vi "GUI_Cameras.vi"(1 "GUIdevice 1":string="HPD_CCD") -> (0 "Image (IMAQ)":T1(plugin-control))   [LabVIEW 2013]
uses:
  Shared/GUI_Template/GUI_master/tcp_new_data_event.ctl
  Shared/GUI_Template/GUI_master/tcp new data cluster.ctl
  color tables/image color table presets.ctl
  Controls/Crosshair type def.ctl
  Controls/IMAQ control.ctl
  <vilib>/vision/Image Controls.llb/IMAQ Image.ctl
  Controls/Image Processing Controls.ctl
  Controls/GUI_running average centroid overlay.ctl
  Controls/Image Analysis Controls.ctl
  <vilib>/Utility/miscctls.llb/LVRectTypeDef.ctl
  <userlib>/_OpenG.lib/comparison/comparison.llb/Boolean Changed__ogtk.vi
  <vilib>/vision/NI_Vision_Development_Module.lvlib
panel:
  in  "stop":bool
  in  "Maximize!!":bool
  out "image::1":T1(plugin-control) caption="HPD_CCD"
  out "tcp data event":T2
  in  "Tab Control":T3(tab)
  in  "Max count":T4(ring)
  in  "Size & Tolerance":T5={"X Size"=5, "Y Size"=5, "% Tolerance"=100} {"Y Size" min=1 max=8; "X Size" min=1 max=8}
  in  "Clear ROI":bool caption="draw Xhair"
  in  "Set ROI":bool caption="draw Xhair"
  in  "LowPass":bool
  out "Max Counts":dbl(slide) scale=0.0..256.0
  in  "Color table":T6
  out "Rate (Hz)":sgl
  in  "analysis::1":bool caption="Analysis"
  in  "Scale":bool
  in  "Autoscale":bool
  in  "trigger::1":bool caption="Trigger"
  in  "save::1":bool caption="Save"
  in  "Beep If Sat.":bool
  in  "roi.offsetY::1":u32 caption="ROI:OffsetY" max=1000
  in  "roi.offsetX::1":u32 caption="ROI:OffsetX" max=1288
  in  "roi.height::1":u32 caption="ROI:Height" min=1 max=728
  in  "roi.width::1":u32 caption="ROI.Width" min=1 max=1288
  in  "SpatialCalibration::1":dbl caption="um/pix" min=0.0 max=9999999.0
  in  "Sat Level":sgl=255.0
  in  "triggerdelay::1":dbl caption="Triggerdelay" min=0.0 max=10000000.0
  in  "exposure::1":dbl=0.52 caption="Exposure" min=1e-07 max=5.0
  in  "gain::1":dbl caption="Gain" min=0.0 max=24.0
  in  "scale factor":dbl=2.0 caption="Scale factor"
  out "UDP error message":string caption="Device Errors"
  in  "Crosshair.Label2::1":string="HPD_CCD" caption="CrosshairLabel2"
  in  "Crosshair.Label1::1":string="HPD_CCD" caption="CrosshairLabel1"
  in  "Target2.X::1":dbl caption="Target2X" min=0.0 max=2000.0
  in  "Target2.Y::1":dbl caption="Target2Y" min=0.0 max=2000.0
  in  "draw Xhair 2":bool caption="draw Xhair"
  in  "Target2Size.X::1":dbl=20.0 caption="Size2 x" min=0.0 max=2000.0
  in  "Target2Size.Y::1":dbl=20.0 caption="Size2 y" min=0.0 max=2000.0
  in  "Crosshair 2\nColor":u32(colorbox)=1250067
  in  "Crosshair 2Thickness":i32=1 caption="Crosshair 2\nThickness" min=0 max=2000
  in  "Overlay\nCentroid":T7={"draw Xhair 2"=FALSE, "Size x"=20.0, "Size y"=20.0, "# images to average"=20, "Centroid \nOverlay Color"=13435100} {"# images to average" min=0 max=2000; "Size y" min=0.0 max=2000.0; "Size x" min=0.0 max=2000.0}
  in  "GUI Crosshair":T8={"Draw"=FALSE, "Target"={"x"=0.0, "y"=0.0}, "Size"={"x"=20.0, "y"=20.0}, "Angle"=0.0, "Color"=1250067, "Thickness"=1, "CrosshairLabel"=""} {"Thickness" max=0; "Angle" format="%#_13g"; "Size"."y" min=0.0 max=0.0; "Size"."x" min=0.0 max=0.0}
  in  "Target.X::1":dbl caption="TargetX" min=0.0 max=2000.0
  in  "Target.Y::1":dbl caption="TargetY" min=0.0 max=2000.0
  in  "draw Xhair":bool=TRUE
  in  "TargetSize.X::1":dbl=20.0 caption="Size x" min=2.0 max=3000.0
  in  "TargetSize.Y::1":dbl=20.0 caption="Size y" min=2.0 max=3000.0
  in  "Crosshair\nColor":u32(colorbox)=1250067
  in  "Crosshair Thickness":i32=1 caption="Crosshair\nThickness" min=0 max=2000
  out "2ndmomW0y45::1":dbl caption="2ndmomW0y45" min=0.0 max=999999.0
  out "2ndmomW0x45::1":dbl caption="2ndmomW0x45" min=0.0 max=999999.0
  out "2ndmomW0y::1":dbl caption="2ndmomW0y" min=0.0 max=999999.0
  in  "Tab Control 2":enum32{"Mean", "Histogram", "Lineout"}(tab)
  out "Chart":dbl[][](graph)
  out "histogram":T9(graph)
  out "Mean Value":sgl format="%.2f"
  out "lineout":cluster{"x0":sgl, "dx":sgl, "Pixels Line":sgl[]}(graph)
  in  "GUI_Analysis":bool
  out "FWHMx (um)":dbl
  out "FWHMy (um)":dbl
  out "2ndmomW0x::1":dbl caption="2ndmomW0x" min=0.0 max=999999.0
  in  "FWHMx::1":dbl caption="FWHMx" min=0.0 max=999999.0
  in  "FWHMy::1":dbl caption="FWHMy" min=0.0 max=999999.0
  in  "centroidx::1":dbl caption="Centroidx" min=0.0 max=0.0
  in  "centroidy::1":dbl caption="Centroidy" min=0.0 max=0.0
  out "meancounts::1":dbl caption="MeanCounts" min=0.0 max=999999999.0
  in  "maxcounts::1":dbl caption="MaxCounts" min=0.0 max=999999999.0
  in  "localsavingpath::1":path caption="LocalSavingPath"
  in  "Hide controls":bool
  out "Current State":string
  # "Mean"
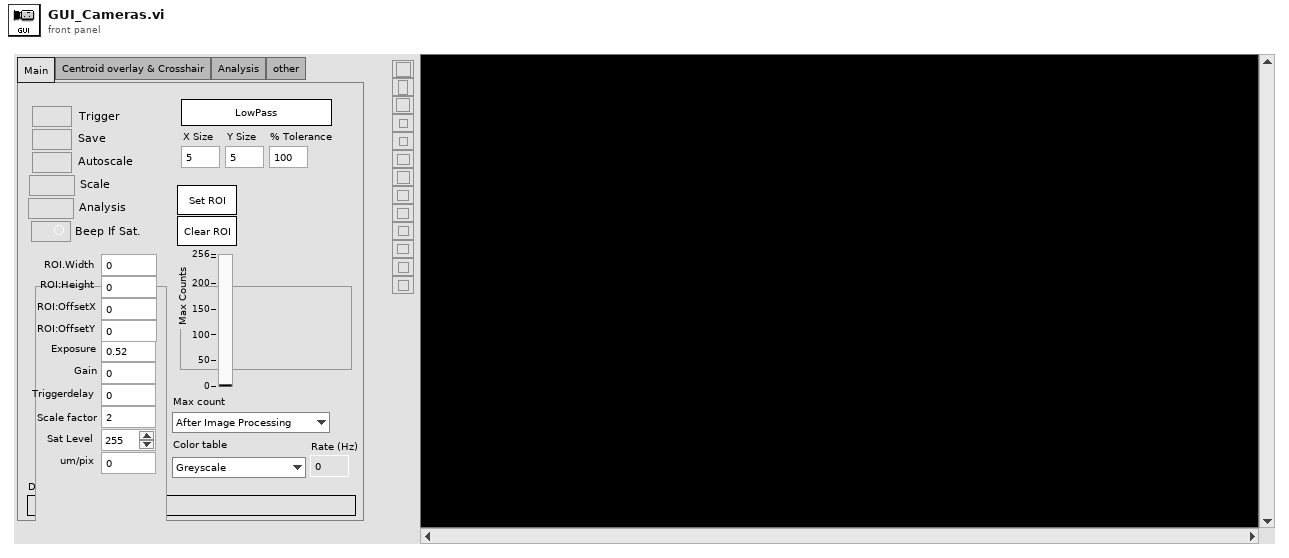
[diagram p1: front panel]
types:
  T1 = typedef "IMAQ Image.ctl" = refnum<image>
  T2 = typedef "tcp_new_data_event.ctl" = refnum<user-event>
  T3 = enum32{"Main", "Centroid overlay & Crosshair", "Analysis", "other"}
  T4 = enum16{"After Image Processing", "Before Image Processing"}
  T5 = cluster{"X Size":i32, "Y Size":i32, "% Tolerance":i32}
  T6 = typedef "image color table presets.ctl" = enum16{"Greyscale", "Binary", "Gradient", "Rainbow", "Temperature", "enhance low", "blue yellow red", "BYR enhance low", "white blue yellow", "BWR enhance low", "make a new one"}
  T7 = cluster{"draw Xhair 2":bool, "Size x":dbl, "Size y":dbl, "# images to average":i32, "Centroid \nOverlay Color":u32}
  T8 = typedef "Crosshair type def.ctl" = cluster{"Draw":bool, "Target":cluster{"x":dbl, "y":dbl}, "Size":cluster{"x":dbl, "y":dbl}, "Angle":dbl, "Color":u32, "Thickness":u8, "CrosshairLabel":string}
  T9 = cluster{"Starting Value":sgl, "Incremental Value":sgl, "Histogram":u32[]}
  T10 = enum32{"Invalid", "Standard", "Closed", "Hidden", "Minimized", "Maximized"}
  T11 = enum32{"invalid app kind", "Development System", "Run Time System", "Student Edition", "Embedded LabVIEW", "Evaluation", "Custom"}
  T12 = typedef "tcp new data cluster.ctl" = cluster{"EventEnum":enum16{"new data", "connection status update"}, "Device name":string}
  T13 = typedef "GUI_running average centroid overlay.ctl" = cluster{"CentroidX array":dbl[], "CentroidY array":dbl[], "CentroidX":dbl, "CentroidY":dbl, "# images to average":i32, "Crosshair":T8}
  T14 = cluster{"2ndmomW0y45::1":dbl, "2ndmomW0x45::1":dbl, "2ndmomW0y::1":dbl, "2ndmomW0x::1":dbl}
  T15 = cluster{"SpatialCalibration":dbl, "FWHMx":dbl, "FWHMy":dbl, "Analysis":bool}
  T16 = cluster{"LowPass":bool, "Size & Tolerance":cluster{"X Size":i32, "Y Size":i32, "% Tolerance":i32}}
  T17 = cluster{"Global Rectangle":i32[], "Contours":cluster{"Contour Type":u32, "ROI Type":u32, "Points":i32[]}[]}
  T18 = typedef "IMAQ Rectangle" = cluster{"Left":i32, "Top":i32, "Right":i32, "Bottom":i32, "Rotation":dbl}
  T19 = typedef "IMAQ control.ctl" = cluster{"Image SM":T1, "valid image":bool, "X resolution":i32, "Y resolution":i32, "Image Area":cluster{"Width":u32, "Height":u32}, "zoom to fit":bool, "Image Center":cluster{"X":u32, "Y":u32}, "Max count":dbl}
  T20 = typedef "Image Processing Controls.ctl" = cluster{"Crosshair IN":T8, "Autoscale":bool, "Scale":cluster{"scale factor":dbl, "Scale":bool}, "Lowpass IN":cluster{"LowPass":bool, "Size & Tolerance":cluster{"X Size":i32, "Y Size":i32, "% Tolerance":i32}}, "Image":T1, "GUI_centroid overlay":T13, "GUI Crosshair":T8, "Crosshair2 IN":T8}
  T21 = typedef "Image Analysis Controls.ctl" = cluster{"Analysis":cluster{"IN":cluster{"SpatialCalibration":dbl, "FWHMx":dbl, "FWHMy":dbl, "Analysis":bool}, "OUT":cluster{"FWHMx (um)":dbl, "FWHMy (um)":dbl}}, "Histogram OUT":cluster{"histogram":cluster{"Starting Value":sgl, "Incremental Value":sgl, "Histogram":u32[]}, "Mean Value Graph":sgl, "Mean Value":sgl}, "Lineout":cluster{"IN":cluster{"ROI":cluster{"Global Rectangle":i32[], "Contours":cluster{"Contour Type":u32, "ROI Type":u32, "Points":i32[]}[]}}, "OUT":cluster{"lineout":cluster{"x0":sgl, "dx":sgl, "Pixels Line":sgl[]}, "Centroid":cluster{"X Centroid":sgl, "Y Centroid":sgl}, "Max Counts":cluster{"Max":sgl, "Color":u32}}}, "Image":T1, "variables":cluster{"2ndmomW0y45::1":dbl, "2ndmomW0x45::1":dbl, "2ndmomW0y::1":dbl, "2ndmomW0x::1":dbl}}
  T22 = typedef "LVRectTypeDef.ctl" = cluster{"Left":i16, "Top":i16, "Right":i16, "Bottom":i16}
  T23 = cluster{"Core":cluster{"Current VI Reference":refnum<vi>, "Close Panel on Exit?":bool}, "tcp connections":refnum<k5>[], "subscribe messages":string[], "Image Data":T19, "Image Process":T20, "Image Analysis":T21, "FP":cluster{"size":T22, "Resize Image":bool}, "Max count":dbl, "Max count before Image Processing":dbl, "Supergui":cluster{"image::1":T1, "STOP queue":refnum<queue>, "SuperGUI ref":refnum<vi>}, "Graph":dbl[][], "New Image":T1, "All Devices":string[]}
  T24 = typedef "Image Type" = u32
  T25 = cluster{"image::1":T1, "STOP queue":refnum<queue>, "SuperGUI ref":refnum<vi>}
  T26 = cluster{"Current VI Reference":refnum<vi>, "Close Panel on Exit?":bool}
  T27 = cluster{"histogram":u32[], "Minimal Value":sgl, "Maximal Value":sgl, "Starting Value":sgl, "Interval Width":sgl, "Mean Value":sgl, "Standard  Variation":sgl, "Area (pixels)":i32}
  T28 = cluster{"TargetSize.X::1":dbl, "TargetSize.Y::1":dbl}
  T29 = cluster{"Target2Size.X::1":dbl, "Target2Size.Y::1":dbl}
  T30 = cluster{"lineout":cluster{"x0":sgl, "dx":sgl, "Pixels Line":sgl[]}, "Centroid":cluster{"X Centroid":sgl, "Y Centroid":sgl}, "Max Counts":cluster{"Max":sgl, "Color":u32}}
  T31 = cluster{"histogram":cluster{"Starting Value":sgl, "Incremental Value":sgl, "Histogram":u32[]}, "Mean Value Graph":sgl, "Mean Value":sgl}
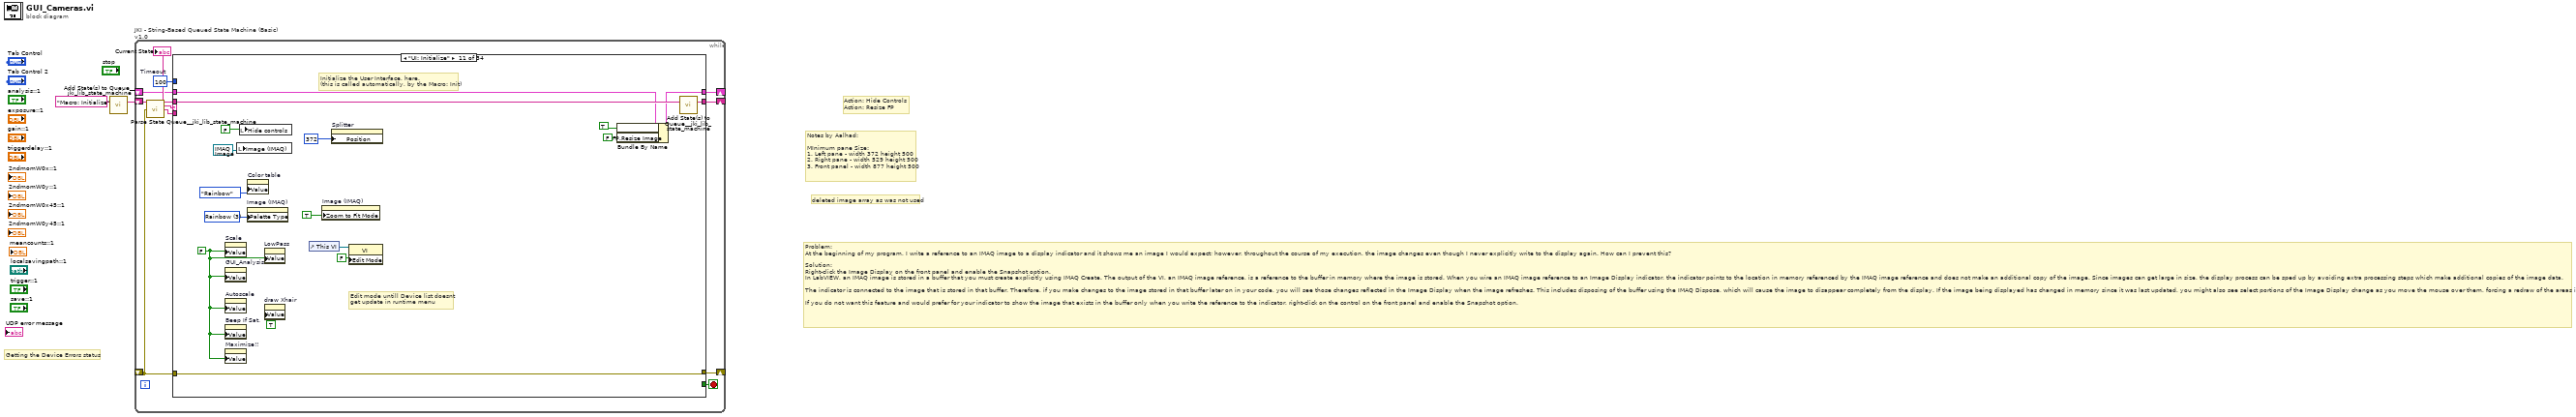
[diagram p0: block diagram]
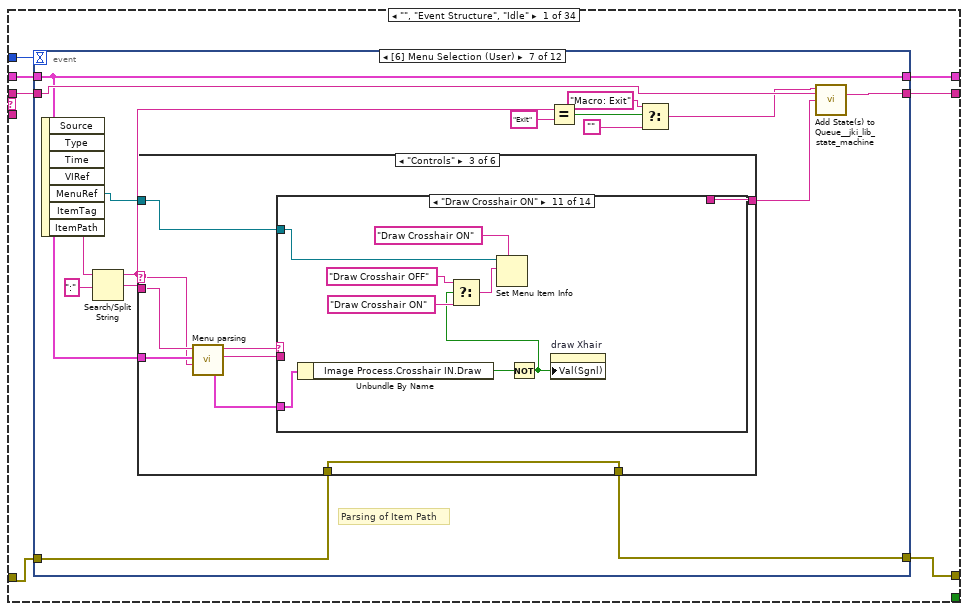
[diagram p2: hidden frame]
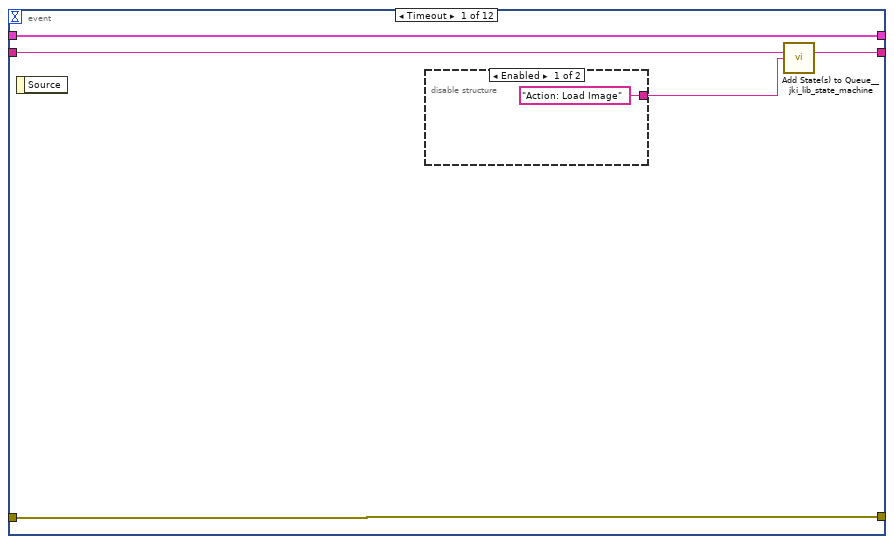
[diagram p3: hidden frame]
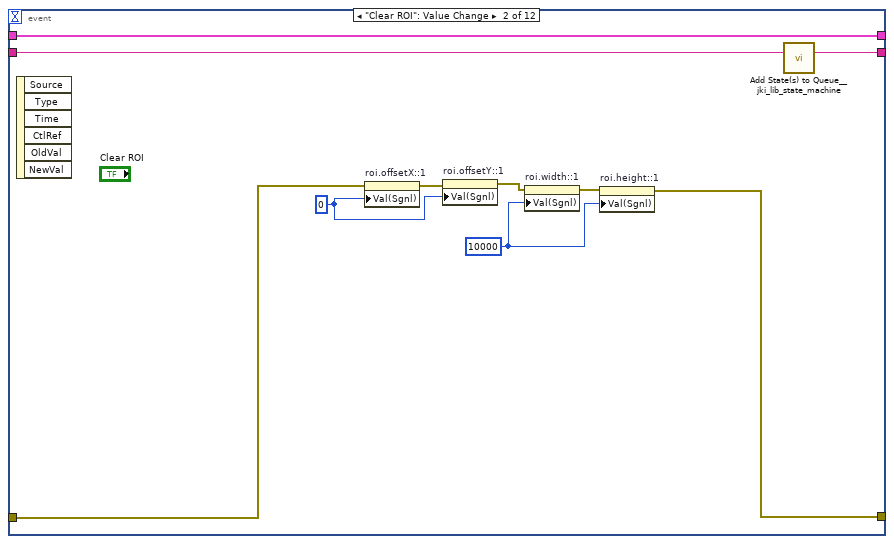
[diagram p5: hidden frame]
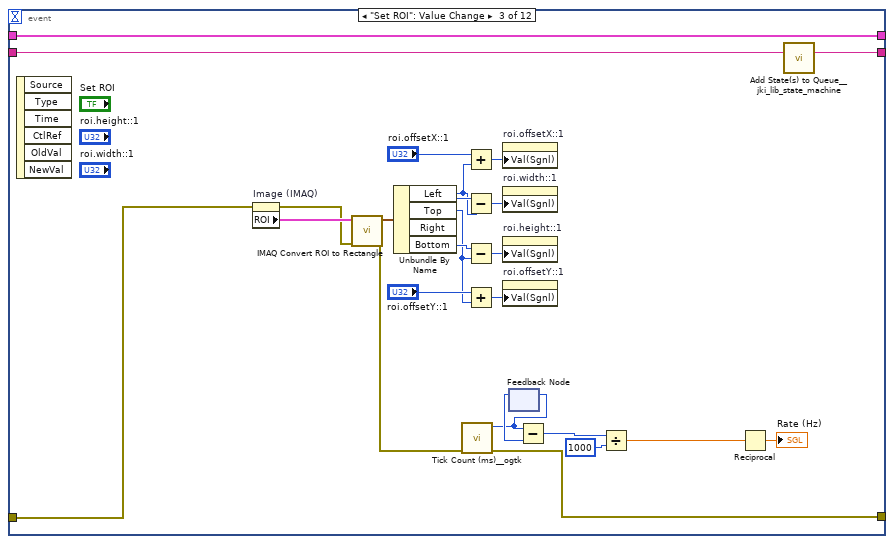
[diagram p6: hidden frame]
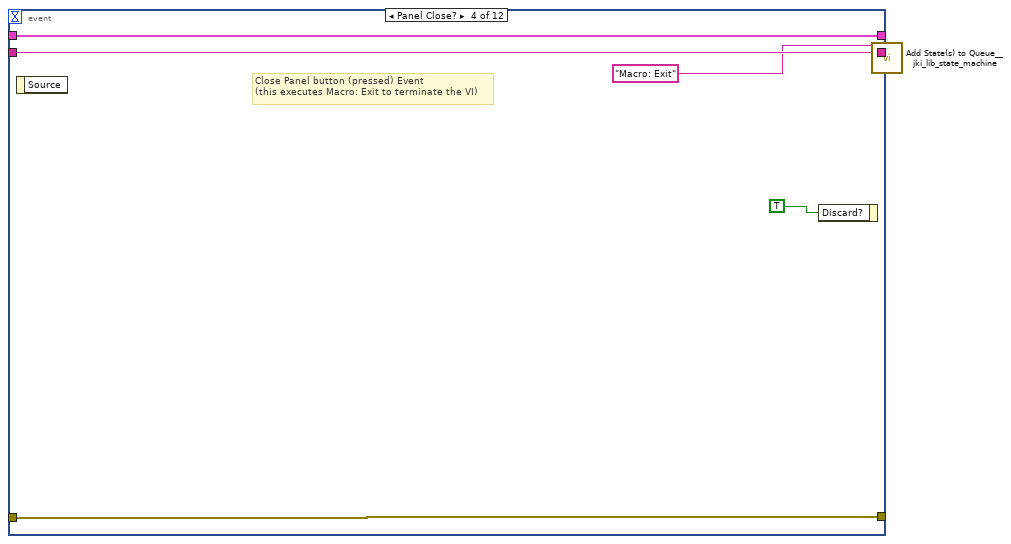
[diagram p7: hidden frame]
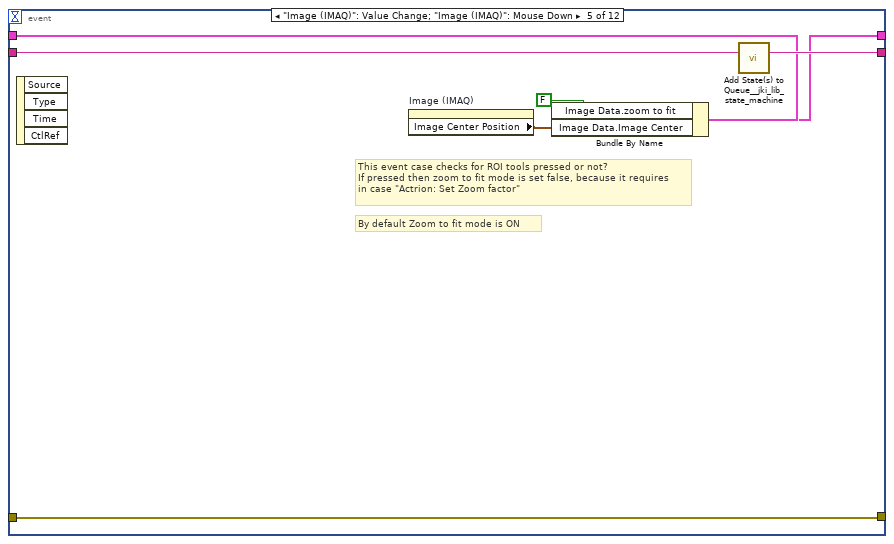
[diagram p8: hidden frame]
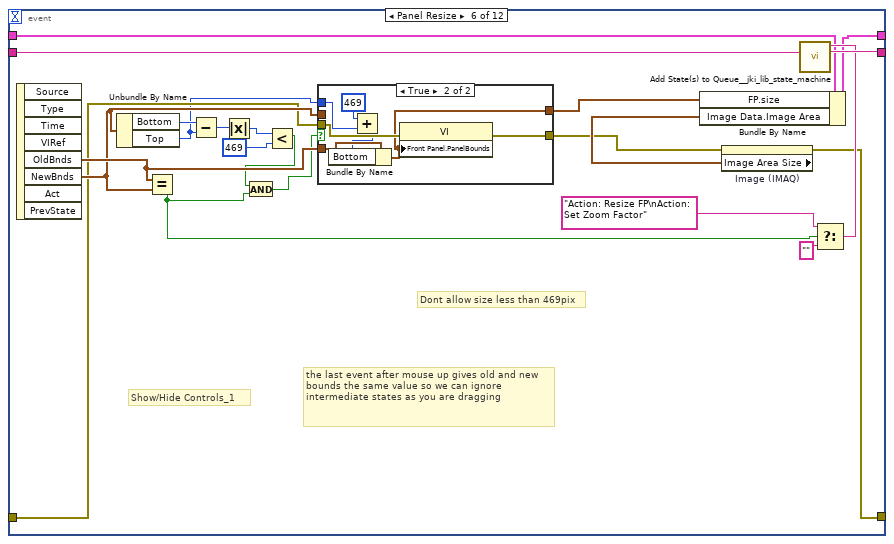
[diagram p9: hidden frame]
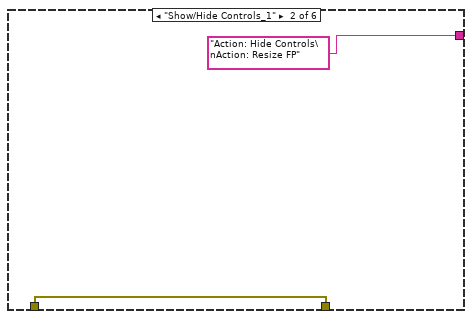
[diagram p12: hidden frame]
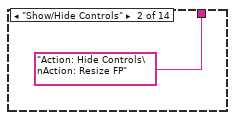
[diagram p14: hidden frame]
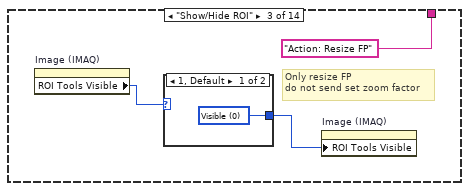
[diagram p15: hidden frame]
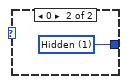
[diagram p16: hidden frame]
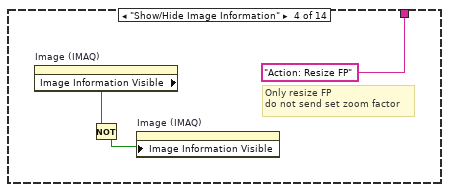
[diagram p17: hidden frame]
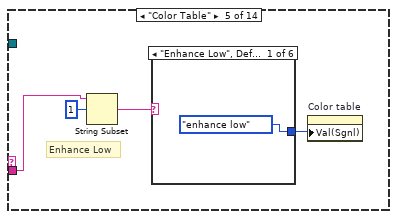
[diagram p18: hidden frame]
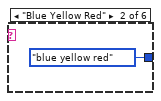
[diagram p19: hidden frame]
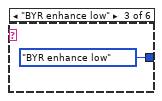
[diagram p20: hidden frame]
diagram:
  # "Getting the Device Errors status"
  # "Notes by Aalhad:\n\nMInimum pane Size:\n1. Left pane - width 372 height 500\n2. Right pane - width 529 height 500\n3. Front panel - width 877 height 500"
  # "deleted image array as was not used"
  # "Problem: \nAt the beginning of my program, I write a reference to an IMAQ image to a display indicator and it shows me an image I would expect; however, throughout the course of my execution, the image changes even though I never explicitly write to the display again. How can I prevent this?\n\nSolution: \nRight-click the Image Display on the front panel and enable the Snapshot option.\nIn LabVIEW, an IMAQ image is stored in a buffer that you must create explicitly using IMAQ Create. The output of the VI, an IMAQ image reference, is a reference to the buffer in memory where the image is stored. When you wire an IMAQ image reference to an Image Display indicator, the indicator points to the location in memory referenced by the IMAQ image reference and does not make an additional copy of the image. Since images can get large in size, the display process can be sped up by avoiding extra processing steps which make additional copies of the image data.\n\nThe indicator is connected to the image that is stored in that buffer. Therefore, if you make changes to the image stored in that buffer later on in your code, you will see those changes reflected in the Image Display when the image refreshes. This includes disposing of the buffer using the IMAQ Dispose, which will cause the image to disappear completely from the display. If the image being displayed has changed in memory since it was last updated, you might also see select portions of the Image Display change as you move the mouse over them, forcing a redraw of the areas it passes through.\n\nIf you do not want this feature and would prefer for your indicator to show the image that exists in the buffer only when you write the reference to the indicator, right-click on the control on the front panel and enable the Snapshot option."
  # "Action: Hide Controls\nAction: Resize FP"
  n1 = call <vilib>:"Add State(s) to Queue__jki_lib_state_machine.vi"("State(s) in (\"\")"="Macro: Initialize") -> ("States Out"=w2:string)  [unwired: 14 in]
  n2 = while "JKI - String-Based Queued State Machine (Basic) v1.0" {
    shift-right: [w6] -> _
    shift-left: _ -> [w5]
    shift-right: [w9] -> _
    shift-left: _ -> [w3]
    shift-right: [w8] -> _
    shift-left: w2 -> [w10]
    stop <- w7 stop-if-true
    w4 = 100  # Timeout
    n3 = call <vilib>:"Parse State Queue__jki_lib_state_machine.vi"("State Queue"=w10, "Error In (no error)"=w3) -> ("Remaining States"=w12:string, "Current State"=w13:string, "Arguments"=w11:string)  [unwired: 11 in]
    "Current State" <- w13
    n4 = case shown="\"UI: Initialize\"" w13 {
      selector: w13 -> [_ _ w302 _ _ _ _ _ _ _ _ _ _ _ _ _ _ _ _ _ _ _ _ _ _ _ _ _ _ _ _ _ _ _]
      tunnel: w12 -> [w20 w301 w306 w324 w332 w347 w351 w376 w385 w392 w409 w421 w426 w462 w487 w518 w540 w550 w585 w590 w595 w607 w611 w632 w646 w687 w713 w783 w797 w818 w840 w856 w874 w899]
      tunnel: w11 -> [_ _ _ _ _ _ _ _ _ _ _ _ _ _ _ _ w535 w545 _ _ _ _ _ _ _ _ _ _ _ _ _ _ _ _]
      tunnel: w5 -> [w18 w298 w304 w316 w330 w345 w348 _ w382 w389 w403 w416 w427 w463 w486 w501 w538 w546 w582 w587 w592 w605 w608 w616 w653 w686 w717 w743 w795 w810 w819 w857 w871 w888]
      tunnel: [w17 w299 w308 w321 w325 w344 w349 w373 w379 w390 w407 w410 w424 w459 w482 w505 w536 w547 w583 w588 w593 w599 w609 w618 w647 w689 w718 w782 w796 w813 w839 w853 w868 w880] -> w9
      tunnel: w3 -> [w16 w299 w307 w321 w326 w344 w349 w373 w378 w390 w407 w417 w425 w460 w481 w502 w537 w548 w583 w588 w593 w599 w609 w625 w648 w706 w715 w782 w796 w814 w839 w854 w869 w878]
      tunnel: [w19 w300 w305 w323 w331 w346 w350 w375 w384 w391 w408 w421 w426 w462 w487 w518 w539 w549 w584 w589 w594 w606 w610 w631 w645 w688 w713 w783 w797 w818 w840 w856 w874 w898] -> w8
      tunnel: [_ _ _ _ _ TRUE _ _ _ _ _ _ _ _ _ _ _ _ _ _ _ _ _ _ _ _ _ _ _ _ _ _ _ _] -> w7
      tunnel: [w15 w298 w304 w322 w330 w345 w348 w374 w382 w389 w402 w415 w427 w463 w486 w504 w538 w546 w582 w587 w592 w605 w608 w617 w652 w685 w716 w781 w794 w815 w819 w857 w871 w888] -> w6
      tunnel: w4 -> [w14 _ _ _ _ _ _ _ _ _ _ _ _ _ _ _ _ _ _ _ _ _ _ _ _ _ _ _ _ _ _ _ _ _]
      frame "", "Event Structure", "Idle" {
        n5 = event shown="[6] Menu Selection (User)" {
          selector: _ -> [_ _ _ _ _ _ _ _ _ _ _ _]
          dyn-events: _ -> [_ _ _ _ _ _ _ _ _ _ _ _]
          timeout: w14 -> [_ _ _ _ _ _ _ _ _ _ _ _]
          tunnel: w20 -> [w25 w36 w61 w67 w73 w95 w113 w253 w271 w275 w281 w297]
          tunnel: [w24 w35 w60 w66 w74 w96 w111 w252 w270 w275 w281 w297] -> w19
          tunnel: w18 -> [w21 w34 w59 w64 w72 w91 w106 w259 w273 w276 w282 w292]
          tunnel: [w23 w27 w37 w65 w71 w79 w108 w254 w272 w274 w277 w296] -> w17
          tunnel: w16 -> [w23 w28 w38 w65 w71 w80 w109 w255 w272 w274 w278 w296]
          tunnel: [w21 w34 w59 w64 w70 w90 w106 w259 w273 w276 w282 w291] -> w15
          event Timeout {
            n6 = event-data() -> ()  [unwired: 1 in, 1 out]
            n7 = disable-structure shown="Enabled" {
              disable-tunnel: ["Action: Load Image" ("State(s) in Front (\"\")") _] -> w22
              frame Enabled {
              }
              frame Disabled {
              }
            }
            n8 = call <vilib>:"Add State(s) to Queue__jki_lib_state_machine.vi"("State(s) in (\"\")"=w25, "State(s) at Back (\"\")"=w22) -> ("States Out"=w24:string)  [unwired: 13 in]
          }
          event "Clear ROI": Value Change {
            w31 = 10000
            w33 = 0
            n9 = event-data() -> ()  [unwired: 1 in, 6 out]
            n10 = property on="roi.offsetX::1" class="DigNum (strict)"(error in=w28, "Val(Sgnl)"=w33) -> (error out=w32:errorcluster)  [unwired: 1 in, 1 out]
            n11 = property on="roi.offsetY::1" class="DigNum (strict)"(error in=w32, "Val(Sgnl)"=w33) -> (error out=w30:errorcluster)  [unwired: 1 in, 1 out]
            n12 = property on="roi.width::1" class="DigNum (strict)"(error in=w30, "Val(Sgnl)"=w31) -> (error out=w29:errorcluster)  [unwired: 1 in, 1 out]
            n13 = property on="roi.height::1" class="DigNum (strict)"(error in=w29, "Val(Sgnl)"=w31) -> (error out=w27:errorcluster)  [unwired: 1 in, 1 out]
            n14 = call <vilib>:"Add State(s) to Queue__jki_lib_state_machine.vi"("State(s) in (\"\")"=w36) -> ("States Out"=w35:string)  [unwired: 14 in]
          }
          event "Set ROI": Value Change {
            n15 = event-data() -> ()  [unwired: 1 in, 6 out]
            n16 = property on="Image (IMAQ)" class="ImageControl"(error in=w38) -> (error out=w40:errorcluster, "ROI"=w57:T17)  [unwired: 1 in, 1 out]
            n17 = call "IMAQ Convert ROI to Rectangle"("error in (no error)"=w40, "ROI Descriptor"=w57) -> ("error out"=w39:errorcluster, "Rectangle"=w58:T18)  [unwired: 7 in]
            n18 = Unbundle By Name(w58) -> ("Left"=w51:i32, "Top"=w48:i32, "Right"=w52:i32, "Bottom"=w49:i32)
            n19 = call <userlib>:"Tick Count (ms)__ogtk.vi"("error in (no error)"=w39) -> ("error out"=w37:errorcluster, "millisecond timer value"=w45:u32)  [unwired: 9 in]
            n20 = Add(x="roi.offsetX::1", y=w51) -> (x+y=w55:u32)
            n21 = Subtract(x=w52, y=w51) -> (x-y=w50:i32)
            n22 = Subtract(x=w49, y=w48) -> (x-y=w47:i32)
            n23 = Add(x="roi.offsetY::1", y=w48) -> (x+y=w53:u32)
            n24 = property on="roi.offsetX::1" class="DigNum (strict)"("Val(Sgnl)"=w55) -> ()  [unwired: 2 in, 2 out]
            n25 = property on="roi.width::1" class="DigNum (strict)"("Val(Sgnl)"=w50) -> ()  [unwired: 2 in, 2 out]
            n26 = property on="roi.height::1" class="DigNum (strict)"("Val(Sgnl)"=w47) -> ()  [unwired: 2 in, 2 out]
            n27 = property on="roi.offsetY::1" class="DigNum (strict)"("Val(Sgnl)"=w53) -> ()  [unwired: 2 in, 2 out]
            n28 = feedback #1() -> (w46:u32)  [unwired: 1 in]
            n29 = feedback-in #1(w45) -> ()
            n30 = Subtract(x=w45, y=w46) -> (x-y=w44:u32)
            n31 = Divide(x=w44, y=u32 1000) -> (x/y=w42:dbl)
            n32 = Reciprocal(x=w42) -> (1/x=→"Rate (Hz)":dbl)
            n33 = call <vilib>:"Add State(s) to Queue__jki_lib_state_machine.vi"("State(s) in (\"\")"=w61) -> ("States Out"=w60:string)  [unwired: 14 in]
          }
          event Panel Close? {
            # "Close Panel button (pressed) Event\n(this executes Macro: Exit to terminate the VI)"
            n34 = event-data() -> ()  [unwired: 1 in, 1 out]
            n35 = event-data("Discard?"=TRUE) -> ()  [unwired: 1 in, 1 out]
            n36 = call <vilib>:"Add State(s) to Queue__jki_lib_state_machine.vi"("State(s) in Front (\"\")"="Macro: Exit", "State(s) in (\"\")"=w67) -> ("States Out"=w66:string)  [unwired: 13 in]
          }
          event "Image (IMAQ)": Value Change; "Image (IMAQ)": Mouse Down {
            # "By default Zoom to fit mode is ON"
            # "This event case checks for ROI tools pressed or not?\nIf pressed then zoom to fit mode is set false, because it requires\nin case \"Actrion: Set Zoom factor\""
            n37 = event-data() -> ()  [unwired: 1 in, 4 out]
            n38 = property on="Image (IMAQ)" class="ImageControl"() -> ("Image Center Position"=w69:cluster{"X":u32, "Y":u32})  [unwired: 2 in, 2 out]
            n39 = Bundle By Name(cluster=w72, "Image Data.zoom to fit"=FALSE, "Image Data.Image Center"=w69) -> (w70:T23)
            n40 = call <vilib>:"Add State(s) to Queue__jki_lib_state_machine.vi"("State(s) in (\"\")"=w73) -> ("States Out"=w74:string)  [unwired: 14 in]
          }
          event Panel Resize {
            # "Dont allow size less than 469pix"
            # "Show/Hide Controls_1"
            # "the last event after mouse up gives old and new bounds the same value so we can ignore intermediate states as you are dragging"
            n41 = event-data() -> ("OldBnds"=w84:T22, "NewBnds"=w82:T22)  [unwired: 1 in, 6 out]
            n42 = Unbundle By Name(w82) -> ("Bottom"=w88:i16, "Top"=w76:i16)
            n43 = Equal?(x=w84, y=w82) -> (x = y?=w75:bool)
            n44 = Subtract(x=w88, y=w76) -> (x-y=w87:i16)
            n45 = Absolute Value(x=w87) -> (abs(x)=w86:i16)
            n46 = Less?(x=w86, y=i16 469) -> (x < y?=w78:bool)
            n47 = And(x=w78, y=w75) -> (x .and. y?=w77:bool)
            n48 = case shown="True" w77 {
              tunnel: w84 -> [_ w103]
              tunnel: [w98 w99] -> w83
              tunnel: w82 -> [w98 _]
              tunnel: [w97 w105] -> w81
              tunnel: w80 -> [w97 w104]
              tunnel: w76 -> [_ w102]
              frame False {
              }
              frame True {
                n49 = Add(x=i16 469 ("y"), y=w102) -> (x+y=w100:i16)
                n50 = Bundle By Name(cluster=w103, "Bottom"=w100) -> (w99:T22)
                n51 = property class="VI"(error in=w104, "Front Panel.PanelBounds"=w99) -> (error out=w105:errorcluster)  [unwired: 1 in, 1 out]
              }
            }
            n52 = property on="Image (IMAQ)" class="ImageControl"(error in=w81) -> (error out=w79:errorcluster, "Image Area Size"=w89:cluster{"Width":u32, "Height":u32})  [unwired: 1 in, 1 out]
            n53 = Bundle By Name(cluster=w91, "FP.size"=w83, "Image Data.Image Area"=w89) -> (w90:T23)
            n54 = Select(t="Action: Resize FP\nAction: Set Zoom Factor" ("State(s) in Front (\"\")"), s=w75, f="" ("t")) -> (s? t:f=w92:string)
            n55 = call <vilib>:"Add State(s) to Queue__jki_lib_state_machine.vi"("State(s) in Front (\"\")"=w92, "State(s) in (\"\")"=w95) -> ("States Out"=w96:string)  [unwired: 13 in]
          }
          event Menu Selection (User) {
            # "Parsing of Item Path"
            n56 = event-data() -> ("MenuRef"=w119:refnum<k9>, "ItemPath"=w121:string)  [unwired: 1 in, 5 out]
            n57 = Search/Split String(string=w121, search string/char (-)=":") -> (substring before match=w110:string, match + rest of string=w118:string)  [unwired: 1 in, 1 out]
            n58 = case shown="\"Controls\"" w110 {
              selector: w110 -> [_ _ w125 w226 _ _]
              tunnel: w118 -> [_ _ w131 w231 _ _]
              tunnel: w119 -> [_ _ w132 _ _ _]
              tunnel: w106 -> [_ _ w128 w225 _ _]
              tunnel: w109 -> [w122 w124 w127 w230 w238 w241]
              tunnel: [w122 w124 w127 w229 w238 w240] -> w108
              tunnel: [_ "Action: Hide Controls\nAction: Resize FP" w126 "UI: Stop SuperGUI\nUI: Start SuperGUI" _ _] -> w107
              frame "", Default {
              }
              frame "Show/Hide Controls_1" {
              }
              frame "Controls" {
                n59 = call "Menu parsing.vi"("Menu Item"=w125, "ItemPath"=w131) -> ("Item Path 2"=w129:string, "ItemPath"=w130:string)  [unwired: 8 in]
                n60 = case shown="\"Draw Crosshair ON\"" w130 {
                  tunnel: w132 -> [_ _ _ _ _ w155 w161 w174 w175 w184 w200 w208 w216 w223]
                  tunnel: w129 -> [_ _ _ _ w143 _ _ _ _ _ _ _ _ _]
                  tunnel: w128 -> [_ _ _ _ _ _ w160 w173 _ _ w198 w203 w213 _]
                  tunnel: [_ "Action: Hide Controls\nAction: Resize FP" "Action: Resize FP" "Action: Resize FP" _ _ _ _ _ _ _ _ _ _] -> w126
                  frame Default {
                  }
                  frame "Show/Hide Controls" {
                  }
                  frame "Show/Hide ROI" {
                    # "Only resize FP\ndo not send set zoom factor"
                    n61 = property on="Image (IMAQ)" class="ImageControl"() -> ("ROI Tools Visible"=w134:u32)  [unwired: 2 in, 2 out]
                    n62 = case shown="1, Default" w134 {
                      tunnel: [w137 w138] -> w136
                      frame 1, Default {
                        w137 = u32 0 items=["Visible", "Hidden", "Hidden, Use WindTools Palette"] ("ROI Tools Visible")
                      }
                      frame 0 {
                        w138 = u32 1 items=["Visible", "Hidden", "Hidden, Use WindTools Palette"] ("ROI Tools Visible")
                      }
                    }
                    n63 = property on="Image (IMAQ)" class="ImageControl"("ROI Tools Visible"=w136) -> ()  [unwired: 2 in, 2 out]
                  }
                  frame "Show/Hide Image Information" {
                    # "Only resize FP\ndo not send set zoom factor"
                    n64 = property on="Image (IMAQ)" class="ImageControl"() -> ("Image Information Visible"=w140:bool)  [unwired: 2 in, 2 out]
                    n65 = Not(x=w140) -> (.not. x?=w139:bool)
                    n66 = property on="Image (IMAQ)" class="ImageControl"("Image Information Visible"=w139) -> ()  [unwired: 2 in, 2 out]
                  }
                  frame "Color Table" {
                    # "Enhance Low"
                    n67 = String Subset(string=w143, offset (0)=1) -> (substring=w142:string)  [unwired: 1 in]
                    n68 = case shown="\"Enhance Low\", Default" w142 {
                      tunnel: [image_color_table_presets."enhance low" ("Value (Signaling)") image_color_table_presets."blue yellow red" ("Value (Signaling)") image_color_table_presets."BYR enhance low" ("Value (Signaling)") image_color_table_presets."white blue yellow" ("Value (Signaling)") image_color_table_presets."BWR enhance low" ("Value (Signaling)") image_color_table_presets."make a new one" ("Value (Signaling)")] -> w145
                      frame "Enhance Low", Default {
                      }
                      frame "Blue Yellow Red" {
                      }
                      frame "BYR enhance low" {
                      }
                      frame "White Blue Yellow" {
                      }
                      frame "BWR enhance low" {
                      }
                      frame "Make a new one" {
                      }
                    }
                    n69 = property on="Color table" class="Enum (strict)"("Val(Sgnl)"=w145) -> ()  [unwired: 2 in, 2 out]
                  }
                  frame "Maximize ON" {
                    n70 = local read "Maximize!!"() -> (w158:bool)
                    n71 = Not(x=w158) -> (.not. x?=w157:bool)
                    n72 = property on="Maximize!!" class="Bool (strict)"("Val(Sgnl)"=w157) -> ()  [unwired: 2 in, 2 out]
                    n73 = Select(t="Maximize OFF" ("item name"), s=w157, f="Maximize ON" ("item name")) -> (s? t:f=w153:string)
                    n74 = Set Menu Item Info(7:"Maximize ON" ("item tag"), 10:w153, 11:w155) -> ()  [unwired: 4 in, 2 out]
                  }
                  frame "Autoscale ON" {
                    n75 = Unbundle By Name(w160) -> ("Image Process.Autoscale"=w159:bool)
                    n76 = Not(x=w159) -> (.not. x?=w166:bool)
                    n77 = Select(t="Autoscale OFF" ("item name"), s=w166, f="Autoscale ON" ("item name")) -> (s? t:f=w162:string)
                    n78 = property on="Autoscale" class="Bool (strict)"("Val(Sgnl)"=w166) -> ()  [unwired: 2 in, 2 out]
                    n79 = Set Menu Item Info(7:"Autoscale ON" ("item tag"), 10:w162, 11:w161) -> ()  [unwired: 4 in, 2 out]
                  }
                  frame "Scale ON" {
                    n80 = Unbundle By Name(w173) -> ("Image Process.Scale.Scale"=w172:bool)
                    n81 = Not(x=w172) -> (.not. x?=w170:bool)
                    n82 = Select(t="Scale OFF" ("item name"), s=w170, f="Scale ON" ("item name")) -> (s? t:f=w167:string)
                    n83 = property on="Scale" class="Bool (strict)"("Val(Sgnl)"=w170) -> ()  [unwired: 2 in, 2 out]
                    n84 = Set Menu Item Info(7:"Scale ON" ("item tag"), 10:w167, 11:w174) -> ()  [unwired: 4 in, 2 out]
                  }
                  frame "Trigger ON" {
                    n85 = local read "trigger::1"() -> (w177:bool)
                    n86 = Not(x=w177) -> (.not. x?=w176:bool)
                    n87 = case shown="False" w176 {
                      tunnel: w175 -> [w179 w182]
                      frame True {
                        n88 = Set Menu Item Info(7:"Trigger ON" ("item tag"), 10:"Trigger OFF" ("item name"), 11:w179) -> ()  [unwired: 4 in, 2 out]
                      }
                      frame False {
                        n89 = Set Menu Item Info(7:"Trigger ON" ("item tag"), 10:"Trigger ON" ("item name"), 11:w182) -> ()  [unwired: 4 in, 2 out]
                      }
                    }
                    n90 = property on="trigger::1" class="Bool (strict)"("Val(Sgnl)"=w176) -> ()  [unwired: 2 in, 2 out]
                  }
                  frame "Save ON" {
                    n91 = local read "save::1"() -> (w186:bool)
                    n92 = Not(x=w186) -> (.not. x?=w185:bool)
                    n93 = case shown="True" w185 {
                      tunnel: w184 -> [w188 w191]
                      frame True {
                        n94 = Set Menu Item Info(7:"Save ON" ("item tag"), 10:"Save OFF" ("item name"), 11:w188) -> ()  [unwired: 4 in, 2 out]
                      }
                      frame False {
                        n95 = Set Menu Item Info(7:"Save ON" ("item tag"), 10:"Save ON" ("item name"), 11:w191) -> ()  [unwired: 4 in, 2 out]
                      }
                    }
                    n96 = property on="save::1" class="Bool (strict)"("Val(Sgnl)"=w185) -> ()  [unwired: 2 in, 2 out]
                  }
                  frame "Draw Crosshair ON" {
                    n97 = Unbundle By Name(w198) -> ("Image Process.Crosshair IN.Draw"=w197:bool)
                    n98 = Not(x=w197) -> (.not. x?=w194:bool)
                    n99 = Select(t="Draw Crosshair OFF" ("item name"), s=w194, f="Draw Crosshair ON" ("item name")) -> (s? t:f=w193:string)
                    n100 = Set Menu Item Info(7:"Draw Crosshair ON" ("item tag"), 10:w193, 11:w200) -> ()  [unwired: 4 in, 2 out]
                    n101 = property on="draw Xhair" class="Bool (strict)"("Val(Sgnl)"=w194) -> ()  [unwired: 2 in, 2 out]
                  }
                  frame "Low Pass ON" {
                    n102 = Unbundle By Name(w203) -> ("Image Process.Lowpass IN.LowPass"=w202:bool)
                    n103 = Not(x=w202) -> (.not. x?=w204:bool)
                    n104 = Select(t="Low Pass OFF" ("item name"), s=w204, f="Low Pass ON" ("item name")) -> (s? t:f=w201:string)
                    n105 = Set Menu Item Info(7:"Low Pass ON" ("item tag"), 10:w201, 11:w208) -> ()  [unwired: 4 in, 2 out]
                    n106 = property on="LowPass" class="Bool (strict)"("Val(Sgnl)"=w204) -> ()  [unwired: 2 in, 2 out]
                  }
                  frame "Analysis ON" {
                    n107 = Unbundle By Name(w213) -> ("Image Analysis.Analysis.IN.Analysis"=w212:bool)
                    n108 = Not(x=w212) -> (.not. x?=w214:bool)
                    n109 = Select(t="Analysis OFF" ("item name"), s=w214, f="Analysis ON" ("item name")) -> (s? t:f=w209:string)
                    n110 = Set Menu Item Info(7:"Analysis ON" ("item tag"), 10:w209, 11:w216) -> ()  [unwired: 4 in, 2 out]
                    n111 = property on="GUI_Analysis" class="Bool (strict)"("Val(Sgnl)"=w214) -> ()  [unwired: 2 in, 2 out]
                  }
                  frame "Beep If Saturation ON" {
                    n112 = local read "Beep If Sat."() -> (w217:bool)
                    n113 = Not(x=w217) -> (.not. x?=w221:bool)
                    n114 = Select(t="Beep If Saturation OFF" ("item name"), s=w221, f="Beep If Saturation ON" ("item name")) -> (s? t:f=w218:string)
                    n115 = Set Menu Item Info(7:"Beep If Saturation ON" ("item tag"), 10:w218, 11:w223) -> ()  [unwired: 4 in, 2 out]
                    n116 = property on="Beep If Sat." class="Bool (strict)"("Val(Sgnl)"=w221) -> ()  [unwired: 2 in, 2 out]
                  }
                }
              }
              frame "Devices" {
                # "#fixed there was race con\ndition here"
                # "#todo stop val sig not nice\nbut current way to gracefully exit\nSuperGUI"
                n117 = Unbundle By Name(w225) -> ("All Devices"=w224:string[])
                n118 = call "Menu parsing.vi"("Menu Item"=w226, "All devices"=w224, "ItemPath"=w231) -> ("ItemPath"=w227:string)  [unwired: 7 in, 1 out]
                n119 = local write "GUIdevice 1"(w227) -> ()
                n120 = flat-sequence {
                  tunnel: [w234] -> w229
                  tunnel: w230 -> [w233]
                  tunnel: w227 -> [w232]
                  frame #0 {
                    # "Set FP title as device name"
                    n121 = control-ref of="This VI"() -> (w237:refnum<vi>)
                    n122 = Concatenate Strings(w232, "_GUI ") -> (w236:string)
                    n123 = property class="VI"(reference=w237, error in=w233, "Front Panel.Title"=w236) -> (error out=w234:errorcluster)  [unwired: 1 out]
                  }
                }
              }
              frame "Exit" {
              }
              frame "Local Saving Path" {
                n124 = control-ref of="localsavingpath::1"() -> (w242:refnum<vi>)
                n125 = property class="Path"(reference=w242, error in=w241) -> (reference out=w244:refnum<vi>, error out=w239:errorcluster, "Value"=w243:path)
                n126 = call "changePath.vi"("Local Saving in (h)"=w243) -> ("change (h)"=w245:bool, "Local Saving out (h)"=w246:path)  [unwired: 9 in]
                n127 = case shown="True" w245 {
                  tunnel: w244 -> [_ w251]
                  tunnel: w246 -> [_ w250]
                  tunnel: [w247 w249] -> w240
                  tunnel: w239 -> [w247 w248]
                  frame False {
                  }
                  frame True {
                    n128 = property class="Path"(reference=w251, error in=w248, "Val(Sgnl)"=w250) -> (error out=w249:errorcluster)  [unwired: 1 out]
                  }
                }
              }
            }
            n129 = Equal?(x=w110, y="Exit") -> (x = y?=w116:bool)
            n130 = Select(t="Macro: Exit", s=w116, f="") -> (s? t:f=w112:string)
            n131 = call <vilib>:"Add State(s) to Queue__jki_lib_state_machine.vi"("State(s) in Front (\"\")"=w112, "State(s) in (\"\")"=w113, "State(s) at Back (\"\")"=w107) -> ("States Out"=w111:string)  [unwired: 12 in]
          }
          event "Maximize!!": Value Change {
            n132 = event-data() -> ()  [unwired: 1 in, 6 out]
            n133 = property class="VI"(error in=w255) -> (error out=w257:errorcluster, "Front Panel.PanelBounds"=w258:T22)  [unwired: 1 in, 1 out]
            n134 = case shown="True" "Maximize!!" {
              tunnel: w258 -> [w263 w267]
              tunnel: [w263 w267] -> _
              tunnel: [w260 w266] -> w254
              tunnel: w257 -> [w261 w264]
              frame False {
                n135 = property class="VI"(error in=w261, "Front Panel Window:State"=T10."Standard") -> (error out=w260:errorcluster)  [unwired: 1 in, 1 out]
              }
              frame True {
                n136 = property class="VI"(error in=w264, "Front Panel Window:State"=T10."Maximized") -> (error out=w266:errorcluster)  [unwired: 1 in, 1 out]
                n137 = Wait (ms)(milliseconds to wait=u32 200) -> ()  [unwired: 1 out]
              }
            }
            n138 = call <vilib>:"Add State(s) to Queue__jki_lib_state_machine.vi"("State(s) in (\"\")"=w253) -> ("States Out"=w252:string)  [unwired: 14 in]
          }
          event Value Change {
            n139 = event-data() -> ()  [unwired: 1 in, 6 out]
            n140 = call <vilib>:"Add State(s) to Queue__jki_lib_state_machine.vi"("State(s) in Front (\"\")"="Action: Color Table", "State(s) in (\"\")"=w271) -> ("States Out"=w270:string)  [unwired: 13 in]
          }
          event "Beep If Sat.": Value Change {
            n141 = event-data() -> ()  [unwired: 1 in, 6 out]
          }
          event "UDP error message": Value Change {
            # "popup message which is in UDP error massage"
            n142 = event-data() -> ("NewVal"=w279:string)  [unwired: 1 in, 5 out]
            n143 = Empty String/Path?(string/path=w279) -> (empty?=w280:bool)
            n144 = case shown="True" w280 {
              tunnel: w279 -> [w286 _]
              tunnel: w278 -> [w285 w287]
              tunnel: [w284 w287] -> w277
              frame False {
                n145 = call "Popup with timeout.vi"("error"=w285, "timeout"=u32 5000, "message"=w286) -> ("error out"=w284:errorcluster)  [unwired: 8 in]
              }
              frame True {
              }
            }
          }
          event "Overlay\nCentroid": Value Change {
            # "Initialize array of data size"
            n146 = event-data() -> ("NewVal"=w288:T7)  [unwired: 1 in, 5 out]
            n147 = Unbundle By Name(w288) -> ("# images to average"=w293:i32)
            n148 = Initialize Array(0.0 ("element"), w293) -> (w290:dbl[])
            n149 = Initialize Array(0.0 ("element"), w293) -> (w289:dbl[])
            n150 = Bundle By Name(cluster=w292, "Image Process.GUI_centroid overlay.CentroidX array"=w290, "Image Process.GUI_centroid overlay.CentroidY array"=w289) -> (w291:T23)
          }
        }
      }
      frame "---------- Core ----------" {
        # "Do not put any code in this frame.\n(it is a separator no-op)"
        n151 = call <vilib>:"Add State(s) to Queue__jki_lib_state_machine.vi"("State(s) in (\"\")"=w301) -> ("States Out"=w300:string)  [unwired: 14 in]
      }
      frame Default {
        w311 = 42 items=["No error", "Argument error", "Memory is full", "Out of zone", "End of file", "File already open", "Generic file I/O error", "File not found", "File permission error", "Disk is full", "Duplicate path", "Too many files open", "System feature not enabled", "Resource file not found", "Cannot add resource", "Resource not found", "Image not found", "Image memory error", "Pen does not exist", "Config type invalid", "Config token not found", "Config parse error", "Config memory error", "Bad external code format", "Bad external code offset", "External code not present", "Null window", "Destroy window error", "Null menu", "Print aborted", "Bad print record", "Print driver error", "Windows error during printing", "Memory error during printing", "Print dialog error", "Generic print error", "Invalid device refnum", "Device not found", "Device parameter error", "Device unit error", "Cannot open device", "Device call aborted", "Generic error", "Cancelled by user", "Object ID too low", "Object ID too high", "Object not in heap", "Unknown heap", "Unknown object (invalid DefProc)", "Unknown object (DefProc not in table)", "Message out of range", "Invalid (null) method", "Unknown message", "Manager call not supported", "Bad address", "Network operation in progress", "Network operation timed out", "Connection is busy", "Network attribute not supported", "Network error", "Address in use", "System out of memory", "Connection aborted", "Connection refused", "Not connected", "Already connected", "Connection closed", "Initialization error (interapplication manager)", "Bad occurrence", "Wait on unbound occurrence handler", "Occurrence queue overflow", "Datalog type conflict", "Unused", "Unrecognized type (interapplication manager)", "Memory corrupt", "Failed to make temporary DLL", "Old CIN version", "Drag socket not found", "Failed to load drop-object", "Failed to register OLE object", "Failed to release OLE object", "Format specifier type mismatch", "Unknown format specifier", "Too few format specifiers", "Too many format specifiers", "Scan failed", "Newer CIN version", "Error converting to variant", "Runtime menu error", "Password tampered", "Variant attribute not found", "Incompatible variant data type", "Event data is not available", "Event Store is not present", "Occurrence is not found", "Event Queue is not created", "Event info is not available", "Refnum passed is NULL", "Error retrieving Class GUID", "Error retrieving CoClass GUID", "Error retrieving TypeLib GUID.", "Bad built application magic bytes.", "Specific driver is different from the specific driver associated with the Logical Name.", "There is no session opened to the class driver.", "Max Error", "MAX - Error with config objects", "MAX - Error loading configuration", "MAX - Group not supported"]
        # "Current State"
        # "Do not delete, rename, or modify this frame.\n(this is used to capture unhandled states and typos)"
        # "Handle mistyped state name (developer tool)"
        n152 = Format Into String(format string="Software Exception: Unhandled State \"%s\"." ("message"), error in=w307, w302) -> (resulting string=w310:string, error out=w309:errorcluster)  [unwired: 1 in]
        n153 = call <vilib>:"Error Cluster From Error Code.vi"("show call chain? (False)"=TRUE, "error in (no error)"=w309, "error message (\"\")"=w310, "error code (0)"=w311) -> ("error out"=w308:errorcluster)  [unwired: 5 in]
        n154 = call <vilib>:"Add State(s) to Queue__jki_lib_state_machine.vi"("State(s) in (\"\")"=w306) -> ("States Out"=w305:string)  [unwired: 14 in]
      }
      frame "Initialize Core Data" {
        # "Do not delete, rename, or modify this frame.\n(this is used to determine panel behavior on exit)"
        # "originally closed?"
        # "exe?"
        # "If panel starts closed or is an EXE, then close it when we exit"
        n155 = property class="VI"() -> ("Front Panel.Open"=w320:bool)  [unwired: 2 in, 2 out]
        n156 = property class="App"() -> ("App.Kind"=w319:T11)  [unwired: 2 in, 2 out]
        n157 = control-ref of="Current VI Reference"() -> (w314:refnum<vi>)
        n158 = Not(x=w320) -> (.not. x?=w317:bool)
        n159 = Equal?(x=w319, y=T11."Run Time System" ("Application:Kind")) -> (x = y?=w313:bool)
        n160 = Or(x=w317, y=w313) -> (x .or. y?=w315:bool)
        n161 = Bundle By Name(cluster=w316, "Core.Current VI Reference"=w314, "Core.Close Panel on Exit?"=w315) -> (w322:T23)
        n162 = call <vilib>:"Add State(s) to Queue__jki_lib_state_machine.vi"("State(s) in (\"\")"=w324) -> ("States Out"=w323:string)  [unwired: 14 in]
      }
      frame "Error Handler" {
        # "Handle any errors here.\nYou can also output any states to clean-up after errors occur"
        n163 = Unbundle By Name(w326) -> ("code"=w327:i32)
        n164 = Absolute Value(x=w327) -> (abs(x)=w328:i32)
        n165 = case shown="1074396072" w328 {
          tunnel: w326 -> [w334 w336]
          tunnel: [errorcluster {"status"=FALSE, "code"=0, "source"=""} ("error out") w337] -> w325
          frame 0, Default {
            # "Unhandled Error -- Display it"
            # "Clear error"
            # "All other errors"
            n166 = call <vilib>:"General Error Handler.vi"("error in (no error)"=w334) -> ()  [unwired: 10 in, 5 out]
          }
          frame 1074396072 {
            # "Low Pass Error Code (Error occurs when image border size above 20)"
            n167 = One Button Dialog(message="Low pass size is too large. Max supported is 7x7", button name ("OK")="OK") -> (true=w335:bool)
            n168 = case shown="True" w335 {
              tunnel: [w340 errorcluster {"status"=FALSE, "code"=0, "source"=""} ("error out")] -> w337
              tunnel: w336 -> [w340 _]
              frame False {
              }
              frame True {
                # "Clear error"
                n169 = property on="LowPass" class="Bool (strict)"("Value"=FALSE ("LowPass")) -> ()  [unwired: 2 in, 2 out]
              }
            }
          }
        }
        n170 = call <vilib>:"Add State(s) to Queue__jki_lib_state_machine.vi"("State(s) in Front (\"\")"="/* Post Error States", "State(s) in (\"\")"=w332) -> ("States Out"=w331:string)  [unwired: 13 in]
      }
      frame "Exit" {
        # "Do not put any code in this frame.\n(No errors that occur here will be handled.)"
        n171 = call <vilib>:"Add State(s) to Queue__jki_lib_state_machine.vi"("State(s) in (\"\")"=w347) -> ("States Out"=w346:string)  [unwired: 14 in]
      }
      frame "---------- Data ----------" {
        # "Do not put any code in this frame.\n(It is a separator no-op. You can make a copy of this frame to create a new Data frame)"
        n172 = call <vilib>:"Add State(s) to Queue__jki_lib_state_machine.vi"("State(s) in (\"\")"=w351) -> ("States Out"=w350:string)  [unwired: 14 in]
      }
      frame "Data: Initialize" {
        w352 = string[] []  # All Devices
        w355 = T24 0 items=["Grayscale (U8)", "Grayscale (I16)", "Grayscale (SGL)", "Complex (CSG)", "RGB (U32)", "HSL (U32)", "RGB (U64)", "Grayscale (U16)"] ("Image Type")
        (unwired) T1 refnum  # ImageChanged
        w357 = dbl[][] []  # Graph
        w358 = T25 {"image::1"="image::1", "STOP queue"=refnum, "SuperGUI ref"=refnum}  # Supergui
        w359 = 0.0  # Max count before Image Processing
        w361 = 0.0  # Max count
        w362 = cluster{"size":T22, "Resize Image":bool} {"size"={"Left"=0, "Top"=0, "Right"=0, "Bottom"=0}, "Resize Image"=FALSE}  # FP
        w363 = T21 {"Analysis"={"IN"={"SpatialCalibration"=0.0, "FWHMx"=0.0, "FWHMy"=0.0, "Analysis"=FALSE}, "OUT"={"FWHMx (um)"=0.0, "FWHMy (um)"=0.0}}, "Histogram OUT"={"histogram"={"Starting Value"=0.0, "Incremental Value"=0.0, "Histogram"=[]}, "Mean Value Graph"=0.0, "Mean Value"=0.0}, "Lineout"={"IN"={"ROI"={"Global Rectangle"=[], "Contours"=[]}}, "OUT"={"lineout"={"x0"=0.0, "dx"=0.0, "Pixels Line"=[]}, "Centroid"={"X Centroid"=0.0, "Y Centroid"=0.0}, "Max Counts"={"Max"=0.0, "Color"=0}}}, "Image"=refnum, "variables"={"2ndmomW0y45::1"=0.0, "2ndmomW0x45::1"=0.0, "2ndmomW0y::1"=0.0, "2ndmomW0x::1"=0.0}}  # Image Analysis
        w364 = T20 {"Crosshair IN"={"Draw"=FALSE, "Target"={"x"=0.0, "y"=0.0}, "Size"={"x"=0.0, "y"=0.0}, "Angle"=0.0, "Color"=0, "Thickness"=0, "CrosshairLabel"=""}, "Autoscale"=FALSE, "Scale"={"scale factor"=0.0, "Scale"=FALSE}, "Lowpass IN"={"LowPass"=FALSE, "Size & Tolerance"={"X Size"=0, "Y Size"=0, "% Tolerance"=0}}, "Image"=refnum, "GUI_centroid overlay"={"CentroidX array"=[], "CentroidY array"=[], "CentroidX"=0.0, "CentroidY"=0.0, "# images to average"=0, "Crosshair"={"Draw"=FALSE, "Target"={"x"=0.0, "y"=0.0}, "Size"={"x"=0.0, "y"=0.0}, "Angle"=0.0, "Color"=0, "Thickness"=0, "CrosshairLabel"=""}}, "GUI Crosshair"={"Draw"=FALSE, "Target"={"x"=0.0, "y"=0.0}, "Size"={"x"=0.0, "y"=0.0}, "Angle"=0.0, "Color"=0, "Thickness"=0, "CrosshairLabel"=""}, "Crosshair2 IN"={"Draw"=FALSE, "Target"={"x"=0.0, "y"=0.0}, "Size"={"x"=0.0, "y"=0.0}, "Angle"=0.0, "Color"=0, "Thickness"=0, "CrosshairLabel"=""}}  # Image Process
        w367 = T24 0 items=["Grayscale (U8)", "Grayscale (I16)", "Grayscale (SGL)", "Complex (CSG)", "RGB (U32)", "HSL (U32)", "RGB (U64)", "Grayscale (U16)"] ("Image Type")
        w368 = string[] []  # subscribe messages
        w370 = T19 {"Image SM"=refnum, "valid image"=FALSE, "X resolution"=0, "Y resolution"=0, "Image Area"={"Width"=0, "Height"=0}, "zoom to fit"=FALSE, "Image Center"={"X"=0, "Y"=0}, "Max count"=0.0}  # Image Data
        w372 = T26 {"Current VI Reference"=refnum, "Close Panel on Exit?"=FALSE}  # Core
        # "Initialize the shift-register data, here.\n(data names are defined by what you wire into the bundle function)"
        n173 = call "IMAQ Create"("Border Size"=21, "Image Name"="image out", "Image Type"=w367) -> ("New Image"=w365:T1)  [unwired: 2 in, 1 out]
        n174 = call "IMAQ Create"("Border Size"=21, "Image Name"="ImageChanged", "Image Type"=w355) -> ("New Image"=w353:T1)  [unwired: 2 in, 1 out]
        n175 = Bundle By Name(cluster=w370, "Image SM"=w365) -> (w369:T19)
        n176 = Bundle("Core"=w372, "tcp connections"=refnum<k5>[] [], "subscribe messages"=w368, "Image Data"=w369, "Image Process"=w364, "Image Analysis"=w363, "FP"=w362, "Max count"=w361, "Max count before Image Processing"=w359, "Supergui"=w358, "Graph"=w357, "New Image"=w353, "All Devices"=w352) -> (w374:T23)  [unwired: 1 in]
        n177 = call <vilib>:"Add State(s) to Queue__jki_lib_state_machine.vi"("State(s) in (\"\")"=w376) -> ("States Out"=w375:string)  [unwired: 14 in]
      }
      frame "Data: Cleanup" {
        # "Cleanup any data and references, here.\n(this is called automatically, by the Macro: Exit)"
        n178 = Unbundle By Name(w382) -> ("Core.Current VI Reference"=w383:refnum<vi>, "Image Data.Image SM"=w381:T1)  [unwired: 2 out]
        n179 = call "IMAQ Dispose"("Image"=w381, "error in (no error)"=w378) -> ("error out"=w377:errorcluster)  [unwired: 4 in]
        n180 = disable-structure shown="Enabled" {
          disable-tunnel: w383 -> [w388 _]
          disable-tunnel: w377 -> [w387 _]
          disable-tunnel: [w386 _] -> w380
          frame Enabled {
            n181 = Close Reference(reference=w388, error in (no error)=w387) -> (error out=w386:errorcluster)
          }
          frame Disabled {
          }
        }
        n182 = call <vilib>:"Clear Errors.vi"("error in (no error)"=w380) -> ("error out"=w379:errorcluster)  [unwired: 6 in]
        n183 = call <vilib>:"Add State(s) to Queue__jki_lib_state_machine.vi"("State(s) in (\"\")"=w385) -> ("States Out"=w384:string)  [unwired: 14 in]
      }
      frame "---------- UI ----------" {
        # "Do not put any code in this frame.\n(It is a separator no-op. You can make a copy of this frame to create a new UI frame)"
        n184 = call <vilib>:"Add State(s) to Queue__jki_lib_state_machine.vi"("State(s) in (\"\")"=w392) -> ("States Out"=w391:string)  [unwired: 14 in]
      }
      frame "UI: Initialize" {
        w400 = FALSE ("hide controls")
        w395 = u32 3 items=["Grayscale", "Binary", "Gradient", "Rainbow", "Temperature", "User Defined"] ("Palette:Palette Type")
        # "Edit mode untill Device list doesnt \nget update in runtime menu"
        # "Initialize the User Interface, here.\n(this is called automatically, by the Macro: Init)"
        n185 = property on="Scale" class="Bool (strict)"("Value"=w400) -> ()  [unwired: 2 in, 2 out]
        n186 = property on="GUI_Analysis" class="Bool (strict)"("Value"=w400) -> ()  [unwired: 2 in, 2 out]
        n187 = property on="Autoscale" class="Bool (strict)"("Value"=w400) -> ()  [unwired: 2 in, 2 out]
        n188 = property on="Beep If Sat." class="Bool (strict)"("Value"=w400) -> ()  [unwired: 2 in, 2 out]
        n189 = property on="Maximize!!" class="Bool (strict)"("Value"=w400) -> ()  [unwired: 2 in, 2 out]
        n190 = local write "Image (IMAQ)"(T1 refnum ("Image Out")) -> ()
        n191 = local write "Hide controls"(FALSE ("hide controls")) -> ()
        n192 = property on="Image (IMAQ)" class="ImageControl"("Palette Type"=w395) -> ()  [unwired: 2 in, 2 out]
        n193 = property on="Color table" class="Enum (strict)"("Value"=image_color_table_presets."Rainbow" ("Color table")) -> ()  [unwired: 2 in, 2 out]
        n194 = property on="LowPass" class="Bool (strict)"("Value"=w400) -> ()  [unwired: 2 in, 2 out]
        n195 = property on="draw Xhair" class="Bool (strict)"("Value"=TRUE ("draw Xhair")) -> ()  [unwired: 2 in, 2 out]
        n196 = control-ref of="This VI"() -> (w399:refnum<vi>)
        n197 = property on="Image (IMAQ)" class="ImageControl"("Zoom to Fit Mode"=TRUE) -> ()  [unwired: 2 in, 2 out]
        n198 = property on="Splitter" class="Splitter"("Position"=372 ("Splitter Position")) -> ()  [unwired: 2 in, 2 out]
        n199 = property class="VI"(reference=w399, "Edit Mode"=FALSE ("Edit Mode On Open")) -> ()  [unwired: 1 in, 2 out]
        n200 = Bundle By Name(cluster=w403, "Image Data.zoom to fit"=TRUE, "FP.Resize Image"=FALSE) -> (w402:T23)
        n201 = call <vilib>:"Add State(s) to Queue__jki_lib_state_machine.vi"("State(s) in (\"\")"=w409) -> ("States Out"=w408:string)  [unwired: 14 in]
      }
      frame "UI: Update Experiment Lines" {
        n202 = control-ref of="This VI"() -> (w418:refnum<vi>)
        n203 = Current VI's Menubar() -> (w420:refnum<k9>)
        n204 = call "Get list of Experiment Lines.vi"("error in (no error)"=w417, "This vi ref"=w418, "menu reference"=w420) -> ("error out"=w412:errorcluster)  [unwired: 7 in, 1 out]
        n205 = for {
          tunnel: [w423] -> w414 mode=concatenating
          tunnel: string[] ["Photometrics_CH-250_Cam", "Point Grey Camera", "Photometrics Cam", "Manta Camera", "Basler Camera", "AndorCamera", "SVimage", "MagSpecCamera", "MagSpecStitcher"] -> [w422] mode=indexing
          n206 = call "getDevices.vi"("Device Class"=w422) -> ("All Devices"=w423:string[])
        }
        n207 = call <vilib>:"Clear Errors.vi"("error in (no error)"=w412) -> ("error out"=w411:errorcluster)  [unwired: 6 in]
        n208 = call "Add devices to expt line menu.vi"("error in (no error)"=w411, "All Devices"=w414, "menu reference"=w420, "This vi ref"=w418) -> ("error out"=w413:errorcluster)  [unwired: 7 in]
        n209 = Bundle By Name(cluster=w416, "All Devices"=w414) -> (w415:T23)
        n210 = Merge Errors(w413, w412) -> (w410:errorcluster)
      }
      frame "UI: Update Device List" {
        n211 = disable-structure shown="Disabled" {
          disable-tunnel: w425 -> [w431 _]
          disable-tunnel: [w430 _] -> w424
          frame Disabled {
            # "#todo this should be in database"
            n212 = Current VI's Menubar() -> (w441:refnum<k9>)
            n213 = Get Menu Item Info(7:"Devices" ("item tag"), 8:w431, 11:w441) -> (0:w434:errorcluster, 3:w439:refnum<k9>)  [unwired: 5 out]
            n214 = Set Menu Item Info(7:"Devices" ("item tag"), 8:w434, 9:TRUE ("enabled"), 11:w439) -> (0:w435:errorcluster, 3:w437:refnum<k9>)  [unwired: 3 in]
            n215 = for {
              tunnel: [w445] -> w428 mode=concatenating
              tunnel: string[] ["Photometrics_CH-250_Cam", "Point Grey Camera", "Photometrics Cam", "Manta Camera", "Basler Camera", "AndorCamera", "SVimage", "MagSpecCamera"] -> [w444] mode=indexing
              n216 = call "getDevices.vi"("Device Class"=w444) -> ("All Devices"=w445:string[])
            }
            n217 = First Call?() -> (First Call?: T/F=w443:bool)
            n218 = case shown="True" w443 {
              tunnel: w437 -> [_ w451]
              tunnel: w428 -> [_ w450]
              tunnel: w435 -> [w446 w448]
              tunnel: [w446 w447] -> w433
              frame False {
              }
              frame True {
                n219 = for {
                  tunnel: [w458] -> w452
                  tunnel: w450 -> [w456] mode=indexing
                  tunnel: w451 -> [w455]
                  tunnel: [w454] -> w449
                  tunnel: w448 -> [w453]
                  n220 = Insert Menu Items(5:"Devices" ("menu tag"), 6:w453, 7:w456, 8:w456, 9:w455) -> (0:w454:errorcluster, 3:w458:refnum<k9>)  [unwired: 1 in, 1 out]
                }
                n221 = Enable Menu Tracking(2:w449, 4:w452) -> (0:w447:errorcluster)  [unwired: 1 in, 1 out]
              }
            }
            n222 = control-ref of="This VI"() -> (w432:refnum<vi>)
            n223 = property class="VI"(reference=w432, error in=w433, "Edit Mode"=TRUE ("Edit Mode On Open")) -> (error out=w430:errorcluster)  [unwired: 1 out]
          }
          frame Enabled {
          }
        }
      }
      frame "UI: Get Device Name" {
        n224 = First Call?() -> (First Call?: T/F=w461:bool)
        n225 = case shown="True" w461 {
          tunnel: w460 -> [w464 w466]
          tunnel: [w464 w465] -> w459
          frame False {
          }
          frame True {
            n226 = disable-structure "Get Device name from control for vi mode\nand command line arg for exe" shown="RUN_TIME_ENGINE==True" {
              disable-tunnel: w466 -> [_ w468]
              disable-tunnel: [_ w467] -> w465
              frame condition #0 (active) {
                (unwired) "Bella_TopviewCCD" ("Device Name for vi mode")
                (unwired) "HPD_CCD" ("Device Name for vi mode")
                (unwired) "P1-SideView" ("Device Name for vi mode")
              }
              frame condition #1 {
                n227 = control-ref of="This Application"() -> (w473:refnum<vi>)
                n228 = property class="App"(reference=w473) -> ("App.Args"=w472:string[])  [unwired: 1 in, 2 out]
                n229 = Index Array(array=w472, index #1=1 ("index")) -> (element #1=w469:string)  [unwired: 2 in, 2 out]
                n230 = flat-sequence {
                  tunnel: [w476] -> w467
                  tunnel: w468 -> [w475]
                  tunnel: w469 -> [w474]
                  frame #0 {
                    # "Set FP title as device name"
                    n231 = control-ref of="This VI"() -> (w479:refnum<vi>)
                    n232 = Concatenate Strings(w474, "_GUI ") -> (w478:string)
                    n233 = property class="VI"(reference=w479, error in=w475, "Front Panel.Title"=w478) -> (error out=w476:errorcluster)  [unwired: 1 out]
                  }
                }
                n234 = Empty String/Path?(string/path=w469) -> (empty?=w470:bool)
                n235 = case shown="False" w470 {
                  tunnel: w469 -> [w480 _]
                  frame False {
                    n236 = local write "GUIdevice 1"(w480) -> ()
                  }
                  frame True {
                  }
                }
              }
            }
          }
        }
      }
      frame "UI: Stop SuperGUI" {
        n237 = Unbundle By Name(w486) -> ("Supergui.SuperGUI ref"=w484:refnum<vi>, "Supergui.STOP queue"=w485:refnum<queue>)
        n238 = disable-structure shown="Disabled" {
          frame Disabled {
            # "note this is for debugging"
            # "how we have stopped supergui (we should change this eventually)"
            # "kills the vi without doing exit code"
            # "what we usually do"
            # "Elsewhere we pass a queue reference into the dynamically called vis and when parent VI the shutdown code executes it closes the queue reference (destroys the queue). The clones then produce an error (e.g. from Get Queue Status) as the queue no longer exists and that error exits the dynamically called vi. Clones shutdown in this way."
            # "#todo"
            n239 = property on="stop" class="Bool (strict)"("Val(Sgnl)"=TRUE ("Value (Signaling)")) -> (error out=w489:errorcluster)  [unwired: 2 in, 1 out]
            n240 = disable-structure shown="Enabled" {
              disable-tunnel: w489 -> [w493 w494]
              disable-tunnel: [w492 w494] -> w488
              frame Enabled {
                n241 = call <userlib>:"Wait (ms)__ogtk.vi"("error in (no error)"=w493, "milliseconds to wait"=u32 5000) -> ("error out"=w492:errorcluster)  [unwired: 8 in, 1 out]
              }
              frame Disabled {
              }
            }
            n242 = disable-structure shown="Disabled" {
              disable-tunnel: _ -> [w496 _]
              disable-tunnel: w488 -> [w495 _]
              frame Disabled {
                n243 = Close Reference(reference=w496, error in (no error)=w495) -> ()  [unwired: 1 out]
              }
              frame Enabled {
              }
            }
          }
          frame Enabled {
          }
        }
        n244 = Release Queue(queue=w485, error in (no error)=w481) -> (error out=w483:errorcluster)  [unwired: 1 in, 2 out]
        n245 = call-by-ref "Wait On Asynchronous Call"(reference=w484, error in=w483) -> ("error out"=w482:errorcluster)  [unwired: 11 in, 2 out]
      }
      frame "UI: Start SuperGUI" {
        w512 = T24 0 items=["Grayscale (U8)", "Grayscale (I16)", "Grayscale (SGL)", "Complex (CSG)", "RGB (U32)", "HSL (U32)", "RGB (U64)", "Grayscale (U16)"] ("Image Type")
        # "create stop queue for supergui and its clones"
        # "can make an icon"
        # "x100 abort will be dependent on caller VI\nx80 abort will be independent of caller vi, this will abort vi when labview is closed."
        n246 = call "IMAQ Create"("Image Name"="image::1", "Image Type"=w512) -> ("New Image"=w513:T1)  [unwired: 3 in, 1 out]
        "image::1" <- w513
        n247 = disable-structure shown="Enabled" {
          disable-tunnel: w513 -> [w524 w528]
          disable-tunnel: w502 -> [w525 _]
          disable-tunnel: [w524 w527] -> w503
          disable-tunnel: [w523 _] -> w510
          disable-tunnel: [w522 _] -> w509
          disable-tunnel: [w521 _] -> w508
          disable-tunnel: [w520 _] -> w507
          disable-tunnel: [w519 _] -> w506
          frame Enabled {
            # "Network acquire image and controls"
            n248 = control-ref of="This Application"() -> (w521:refnum<vi>)
            n249 = control-ref of="This VI"() -> (w520:refnum<vi>)
            n250 = Create User Event(user event datatype=T12 {"EventEnum"=enum."new data", "Device name"="Device name"} ("New Event"), error in=w525) -> (user event=w522:refnum<user-event>, error out=w523:errorcluster)
            "tcp data event" <- w522
            n251 = Current VI's Menubar() -> (w519:refnum<k9>)
            n252 = register-events(w522) -> ()  [unwired: 2 in, 2 out]
          }
          frame Disabled {
            # "Simulation mode"
            n253 = while {
              shift-right: [w531] -> w527
              shift-left: w528 -> [w532]
              stop <- w529 stop-if-true
              # "This creates an image of a Gaussian beam"
              n254 = call "StopFGV.vi"("Command"=enum16{"set", "get", "init"}."get") -> ("Stop out"=w529:bool)  [unwired: 9 in, 1 out]
              n255 = call "2d Gaussian array.vi"() -> ("Array"=w534:u8[][])  [unwired: 11 in]
              n256 = call "IMAQ ArrayToImage"("Image Pixels (U8)"=w534, "Image"=w532) -> ("Image Out"=w531:T1)  [unwired: 8 in, 1 out]
              n257 = Wait (ms)(milliseconds to wait=u32 1000) -> ()  [unwired: 1 out]
            }
          }
        }
        n258 = vi-ref "GUI_Master_subvi_reentrant_queues.vi"() -> (w499:refnum<vi>)
        n259 = call "supergui create stop queue.vi"() -> ("STOP Queue out"=w500:refnum<queue>)  [unwired: 11 in]
        n260 = property class="VI"(reference=w499) -> ("Path"=w498:path)  [unwired: 1 in, 2 out]
        n261 = Open VI Reference(type specifier VI Refnum (for type only)=refnum<vi> refnum, vi path=w498, options=256, error in (no error)=w502) -> (vi reference=w517:refnum<vi>, error out=w516:errorcluster)  [unwired: 2 in]
        n262 = call-by-ref "Start Asynchronous Call"(reference=w517, error in=w516, "STOP Queue in"=w500, "This Application"=w508, 8:"error in (no error)"=w510, "tcp data event"=w509, "Caller menu reference"=w506, "Caller VI ref"=w507) -> (reference out=w497:refnum<vi>, error out=w505:errorcluster)  [unwired: 5 in, 1 out]
        n263 = Bundle By Name(cluster=w501, "Supergui.image::1"=w503, "Supergui.SuperGUI ref"=w497, "Supergui.STOP queue"=w500) -> (w504:T23)
      }
      frame "UI: Cursor Set" {
        # "Argument"
        # "Set and Unset Cursor Busy.\n(Usage: \"UI: Cursor Set >> Busy|Idle\")"
        n264 = case shown="\"Idle\", Default" w535 {
          tunnel: w537 -> [w542 w544]
          tunnel: [w541 w543] -> w536
          frame "Idle", Default {
            n265 = call <vilib>:"Unset Busy.vi"("error in (no error)"=w542) -> ("error out"=w541:errorcluster)  [unwired: 10 in]
          }
          frame "Busy" {
            n266 = call <vilib>:"Set Busy.vi"("error in (no error)"=w544) -> ("error out"=w543:errorcluster)  [unwired: 9 in, 1 out]
          }
        }
        n267 = call <vilib>:"Add State(s) to Queue__jki_lib_state_machine.vi"("State(s) in (\"\")"=w540) -> ("States Out"=w539:string)  [unwired: 14 in]
      }
      frame "UI: Front Panel State" {
        # "Set Front Panel Open or Closed\n(Usage: \"UI: Front Panel State >> Open|Close\")"
        n268 = disable-structure shown="Enabled" {
          disable-tunnel: w548 -> [w555 _]
          disable-tunnel: [w554 _] -> w547
          disable-tunnel: w546 -> [w553 _]
          disable-tunnel: w545 -> [w551 _]
          frame Enabled {
            # "Argument"
            n269 = Unbundle By Name(w553) -> ("Core.Current VI Reference"=w552:refnum<vi>)
            n270 = case shown="\"Open\", Default" w551 {
              tunnel: w555 -> [w559 w572]
              tunnel: [w561 w573] -> w554
              tunnel: w552 -> [w560 w570]
              frame "Open", Default {
                n271 = property class="VI"(reference=w560, error in=w559) -> (reference out=w557:refnum<vi>, error out=w558:errorcluster, "Front Panel.Open"=w556:bool)
                n272 = case shown="True" w556 {
                  tunnel: [w564 w567] -> w561
                  tunnel: w558 -> [w563 w567]
                  tunnel: w557 -> [w562 _]
                  frame False {
                    n273 = invoke class="VI" method="FP.Open"(reference=w562, error in=w563, "Activate"=TRUE, "State"=T10."Standard") -> (error out=w564:errorcluster)  [unwired: 1 in, 4 out]
                  }
                  frame True {
                  }
                }
              }
              frame "Close" {
                n274 = property class="VI"(reference=w570, error in=w572) -> (reference out=w569:refnum<vi>, error out=w571:errorcluster, "Front Panel.Open"=w568:bool)
                n275 = disable-structure shown="Enabled" {
                  disable-tunnel: [w577 _] -> w573
                  disable-tunnel: w571 -> [w576 _]
                  disable-tunnel: w569 -> [w575 _]
                  disable-tunnel: w568 -> [w574 _]
                  frame Enabled {
                    n276 = case shown="True" w574 {
                      tunnel: [w578 w581] -> w577
                      tunnel: w576 -> [w578 w580]
                      tunnel: w575 -> [_ w579]
                      frame False {
                      }
                      frame True {
                        n277 = invoke class="VI" method="FP.Close"(reference=w579, error in=w580) -> (error out=w581:errorcluster)  [unwired: 1 in, 2 out]
                      }
                    }
                  }
                  frame Disabled {
                  }
                }
              }
            }
          }
          frame Disabled {
          }
        }
        n278 = call <vilib>:"Add State(s) to Queue__jki_lib_state_machine.vi"("State(s) in (\"\")"=w550) -> ("States Out"=w549:string)  [unwired: 14 in]
      }
      frame "---------- Macro ----------" {
        # "Do not put any code in this frame.\n(It is a separator no-op. You can make a copy of this frame to create a new Macro frame)"
        n279 = call <vilib>:"Add State(s) to Queue__jki_lib_state_machine.vi"("State(s) in (\"\")"=w585) -> ("States Out"=w584:string)  [unwired: 14 in]
      }
      frame "Macro: Initialize" {
        w586 = "Data: Initialize\nInitialize Core Data\nUI: Initialize\nUI: Update Experiment Lines\nUI: Update Device List\nUI: Get Device Name\nUI: Start SuperGUI\nUI: Front Panel State >> Open"  # Data: Initialize Initialize Core Data UI: Initialize UI: Update Experiment Lines UI: Update Device List UI: Get Device Name UI: Start SuperGUI UI: Front Panel State >> Open
        # "Initialization Macro\n(This is called once, when the VI starts)"
        n280 = call <vilib>:"Add State(s) to Queue__jki_lib_state_machine.vi"("State(s) in Front (\"\")"=w586, "State(s) in (\"\")"=w590) -> ("States Out"=w589:string)  [unwired: 13 in]
      }
      frame "Macro: valid image" {
        # "Initialization Macro\n(This is called once, when the VI starts)"
        n281 = call <vilib>:"Add State(s) to Queue__jki_lib_state_machine.vi"("State(s) in Front (\"\")"="Action: Resize FP\nAction: Set Zoom Factor\nAction: Read Controls\nAction: Read Controls 2\nAction: Display Image", "State(s) in (\"\")"=w595) -> ("States Out"=w594:string)  [unwired: 13 in]
      }
      frame "Macro: Exit" {
        # "Exit Macro\n(This is called once, when the VI exits)"
        n282 = Unbundle By Name(w605) -> ("Core.Close Panel on Exit?"=w604:bool, "Supergui.image::1"=w597:T1)
        n283 = call "IMAQ Dispose"("Image"=w597) -> ()  [unwired: 5 in, 1 out]
        n284 = Select(t="UI: Front Panel State >> Close", s=w604, f="") -> (s? t:f=w602:string)
        n285 = call <vilib>:"Add State(s) to Queue__jki_lib_state_machine.vi"("State(s) in Front (\"\")"="UI: Stop SuperGUI" ("State(s) in Front (\"\")"), "State(s) in (\"\")"=w602, "State(s) at Back (\"\")"="Data: Cleanup\nExit") -> ("States Out"=w600:string)  [unwired: 12 in]
        n286 = call <vilib>:"Add State(s) to Queue__jki_lib_state_machine.vi"("State(s) in Front (\"\")"=w600, "State(s) in (\"\")"=w607) -> ("States Out"=w606:string)  [unwired: 13 in]
      }
      frame "---------- New Category ----------" {
        # "Template Separator\n(You can make a copy of, or modify, this frame)"
        n287 = call <vilib>:"Add State(s) to Queue__jki_lib_state_machine.vi"("State(s) in (\"\")"=w611) -> ("States Out"=w610:string)  [unwired: 14 in]
      }
      frame "Action: Load Image" {
        w614 = "image::1" ("Image Name")
        # "Max count from actual image"
        # "Is image the same?\nif yes do nothing.\nIf no then go to get image size\nIf size different then \nResize FP and set zoom factor\nIf not don't above either way\nprocess and display image"
        # "Load Image from File"
        n288 = Unbundle By Name(w616) -> ("New Image"=w621:T1, "Image Data.Image SM"=w613:T1)
        n289 = call "IMAQ Histograph"("error in (no error)"=w625, "Image"=w621) -> ("error out"=w628:errorcluster, "Histogram Graph"=w622:T9)  [unwired: 6 in, 2 out]
        n290 = call <vilib>:"Clear Errors.vi"("error in (no error)"=w628) -> ("error out"=w624:errorcluster)  [unwired: 6 in]
        n291 = call "IMAQ Histograph"("error in (no error)"=w624, "Image"=w614) -> ("error out"=w629:errorcluster, "Histogram Graph"=w630:T9)  [unwired: 6 in, 2 out]
        n292 = Not Equal?(x=w630, y=w622) -> (x != y?=w626:bool)
        n293 = call <vilib>:"Clear Errors.vi"("error in (no error)"=w629) -> ("error out"=w623:errorcluster)  [unwired: 6 in]
        n294 = call "IMAQ Copy"("error in (no error)"=w623, "Image Dst"=w621, "Image Src"=w614) -> ("error out"=w619:errorcluster, "Image Dst Out"=w620:T1)  [unwired: 3 in]
        n295 = call "IMAQ Copy"("Image Dst"=w613, "Image Src"=w614) -> ("Image Dst Out"=w612:T1)  [unwired: 4 in, 1 out]
        n296 = case shown="True" w626 {
          tunnel: [_ "Action: Get Image Size"] -> w627
          tunnel: w620 -> [_ w641]
          tunnel: w616 -> [w633 w637]
          tunnel: w619 -> [w634 w639]
          tunnel: [w634 w638] -> w618
          tunnel: [w633 w636] -> w615
          frame False {
          }
          frame True {
            # "image is new"
            n297 = call "IMAQ Histogram"("error in (no error)"=w639, "Image"=w641) -> ("error out"=w638:errorcluster, "Histogram Report"=w640:T27)  [unwired: 8 in]
            n298 = Unbundle By Name(w640) -> ("Maximal Value"=w635:sgl)
            n299 = Bundle By Name(cluster=w637, "Max count"=w635, "Max count before Image Processing"=w635) -> (w636:T23)
          }
        }
        n300 = call <vilib>:"Add State(s) to Queue__jki_lib_state_machine.vi"("State(s) in Front (\"\")"=w627, "State(s) in (\"\")"=w632) -> ("States Out"=w631:string)  [unwired: 13 in]
        n301 = Bundle By Name(cluster=w615, "Image Data.Image SM"=w620, "New Image"=w612) -> (w617:T23)
      }
      frame "Action: Get Image Size" {
        n302 = Unbundle By Name(w653) -> ("Image Data.X resolution"=w655:i32, "Image Data.Y resolution"=w654:i32, "Image Data.Image SM"=w643:T1)
        n303 = case shown="No Error" w648 {
          selector: w648 -> [w663 w683]
          tunnel: [w664 _] -> w651
          tunnel: [w661 _] -> w650
          tunnel: w643 -> [w662 _]
          tunnel: [w657 _] -> w649
          tunnel: [w669 w683] -> w647
          tunnel: [w660 _] -> w644
          tunnel: w655 -> [w668 _]
          tunnel: w654 -> [w667 _]
          frame No Error {
            n304 = call "Get Resolution.vi"("Image"=w662, "error in (no error)"=w663) -> ("X Resolution"=w664:i32, "Y Resolution"=w661:i32, "Image Area:Size:All Elements"=w657:cluster{"Width":u32, "Height":u32}, "valid Image"=w659:bool, "error out"=w656:errorcluster)  [unwired: 9 in]
            n305 = Build Array(w668, w667) -> (w666:i32[])
            n306 = Build Array(w664, w661) -> (w665:i32[])
            n307 = Not Equal?(x=w666, y=w665) -> (x != y?=w658:bool)
            n308 = case shown="True" w659 {
              tunnel: [w670 w677] -> w669
              tunnel: w656 -> [w670 w676]
              tunnel: ["" w672] -> w660
              tunnel: w658 -> [_ w675]
              frame False {
                # "image not valid"
              }
              frame True {
                # "Image valid"
                n309 = case shown="False" w675 {
                  tunnel: [w679 w682] -> w677
                  tunnel: w676 -> [w679 w681]
                  tunnel: ["" "Action: Resize FP\nAction: Set Zoom Factor"] -> w673
                  frame False {
                    # "Image size not changed"
                  }
                  frame True {
                    # "Image res changed"
                    n310 = invoke on="Image (IMAQ)" class="ImageControl" method="FitControlToPane"(error in=w681) -> (error out=w682:errorcluster)  [unwired: 2 in, 2 out]
                  }
                }
                n311 = call <vilib>:"Add State(s) to Queue__jki_lib_state_machine.vi"("State(s) in (\"\")"=w673, "State(s) at Back (\"\")"="Action: Read Controls\nAction: Read Controls 2\nAction: Process Image\nAction: Display Image") -> ("States Out"=w672:string)  [unwired: 13 in]
              }
            }
          }
          frame Error {
          }
        }
        n312 = Bundle By Name(cluster=w653, "Image Data.X resolution"=w651, "Image Data.Y resolution"=w650, "Image Data.Image Area"=w649) -> (w652:T23)
        n313 = call <vilib>:"Add State(s) to Queue__jki_lib_state_machine.vi"("State(s) in Front (\"\")"=w644, "State(s) in (\"\")"=w646) -> ("States Out"=w645:string)  [unwired: 13 in]
      }
      frame "Action: Resize FP" {
        # "Resize FP as per\nthe image size"
        # "Adjust the aspect ration as per the \nresize image height and width"
        # "Aspect ratio"
        # "Resizes Front panel as per the image size. The new vertical size is used to adjust the right panel bounds so that the panel size matches the image aspect ratio"
        n314 = disable-structure shown="Enabled" {
          disable-tunnel: w706 -> [w709 _]
          disable-tunnel: [w708 _] -> w690
          frame Enabled {
            n315 = invoke on="Image (IMAQ)" class="ImageControl" method="FitControlToPane"(error in=w709) -> (error out=w708:errorcluster)  [unwired: 2 in, 2 out]
          }
          frame Disabled {
          }
        }
        n316 = Unbundle By Name(w686) -> ("Image Data.Y resolution"=w692:i32, "Image Data.X resolution"=w691:i32)
        n317 = property on="Image (IMAQ)" class="ImageControl"(error in=w690) -> (error out=w694:errorcluster, "Image Area Height"=w704:u32, "Image Area Width"=w701:u32)  [unwired: 1 in, 1 out]
        n318 = Divide(x=w692, y=w691) -> (x/y=w705:dbl)
        n319 = control-ref of="This VI"() -> (w700:refnum<vi>)
        n320 = property class="VI"(reference=w700, error in=w694) -> (reference out=w698:refnum<vi>, error out=w693:errorcluster, "Front Panel.PanelBounds"=w699:T22)
        n321 = Divide(x=w704, y=w705) -> (x/y=w702:dbl)
        n322 = Subtract(x=w702, y=w701) -> (x-y=w703:dbl)
        n323 = Unbundle By Name(w699) -> ("Right"=w697:i16)
        n324 = To Word Integer(number=w703) -> (16bit integer=w696:i16)
        n325 = Add(x=w697, y=w696) -> (x+y=w695:i16)
        n326 = Bundle By Name(cluster=w699, "Right"=w695) -> (w684:T22)
        n327 = Bundle By Name(cluster=w686, "FP.size"=w684) -> (w685:T23)
        n328 = property class="VI"(reference=w698, error in=w693, "Front Panel.PanelBounds"=w684) -> (error out=w707:errorcluster)  [unwired: 1 out]
        n329 = call <vilib>:"Add State(s) to Queue__jki_lib_state_machine.vi"("State(s) in (\"\")"=w687) -> ("States Out"=w688:string)  [unwired: 14 in]
        n330 = call <vilib>:"Clear Errors.vi"("error in (no error)"=w707) -> ("error out"=w689:errorcluster)  [unwired: 6 in]
      }
      frame "Action: Set Zoom Factor" {
        # "#todo the recenter image position is no longer working"
        # "Changed size of image"
        # "Calcultes zoom factor for image as per the changed size of image"
        n331 = Unbundle By Name(w717) -> ("Image Data.Image Area"=w719:cluster{"Width":u32, "Height":u32}, "Image Data.Image Center"=w712:cluster{"X":u32, "Y":u32}, "Image Data.zoom to fit"=w711:bool)
        n332 = disable-structure shown="Enabled" {
          disable-tunnel: w715 -> [w726 _]
          disable-tunnel: [w725 _] -> w714
          frame Enabled {
            n333 = invoke on="Image (IMAQ)" class="ImageControl" method="FitControlToPane"(error in=w726) -> (error out=w725:errorcluster)  [unwired: 2 in, 2 out]
          }
          frame Disabled {
          }
        }
        n334 = property on="Image (IMAQ)" class="ImageControl"(error in=w714) -> ("Image Area Size"=w723:cluster{"Width":u32, "Height":u32})  [unwired: 1 in, 2 out]
        n335 = Not Equal?(x=w719, y=w723) -> (x != y?=w724:bool)
        n336 = case shown="True" w724 {
          tunnel: w723 -> [_ w733]
          tunnel: w719 -> [_ w732]
          tunnel: [_ w728] -> w722
          frame False {
          }
          frame True {
            n337 = property on="Image (IMAQ)" class="ImageControl"() -> ("ZoomSingle"=w731:cluster{"X":sgl, "Y":sgl})  [unwired: 2 in, 2 out]
            n338 = Divide(x=w733, y=w732) -> (x/y=w729:cluster{"Width":dbl, "Height":dbl})
            n339 = Unbundle(w729) -> ("Height"=w727:dbl)  [unwired: 1 out]
            n340 = Multiply(x=w727, y=w731) -> (x*y=w730:cluster{"X":dbl, "Y":dbl})
            n341 = property on="Image (IMAQ)" class="ImageControl"("ZoomSingle"=w730) -> (error out=w728:errorcluster)  [unwired: 2 in, 1 out]
          }
        }
        n342 = property on="Image (IMAQ)" class="ImageControl"(error in=w722, "Image Center Position"=w712) -> (error out=w720:errorcluster)  [unwired: 1 in, 1 out]
        n343 = property on="Image (IMAQ)" class="ImageControl"(error in=w720, "Zoom to Fit Mode"=w711) -> (error out=w721:errorcluster)  [unwired: 1 in, 1 out]
        n344 = property on="Image (IMAQ)" class="ImageControl"(error in=w721) -> (error out=w718:errorcluster, "Image Area Size"=w710:cluster{"Width":u32, "Height":u32})  [unwired: 1 in, 1 out]
        n345 = Bundle By Name(cluster=w717, "Image Data.Image Area"=w710) -> (w716:T23)
      }
      frame "Action: Read Controls" {
        n346 = Unbundle By Name(w743) -> ("Image Data.Image SM"=w765:T1)
        n347 = Bundle("TargetSize.X::1"="TargetSize.X::1", "TargetSize.Y::1"="TargetSize.Y::1") -> (w760:T28)  [unwired: 1 in]
        n348 = Bundle By Name(cluster=T15 {"SpatialCalibration"=0.0, "FWHMx"=0.0, "FWHMy"=0.0, "Analysis"=FALSE} ("Image Process.Analysis.IN"), "Analysis"="GUI_Analysis", "SpatialCalibration"="SpatialCalibration::1", "FWHMx"="FWHMx::1", "FWHMy"="FWHMy::1") -> (w764:T15)
        n349 = Bundle By Name(cluster=T16 {"LowPass"=FALSE, "Size & Tolerance"={"X Size"=0, "Y Size"=0, "% Tolerance"=0}} ("Image Process.Lowpass IN"), "LowPass"="LowPass", "Size & Tolerance"="Size & Tolerance") -> (w772:T16)
        n350 = Bundle By Name(cluster=cluster{"scale factor":dbl, "Scale":bool} {"scale factor"=0.0, "Scale"=FALSE} ("Image Process.Scale"), "scale factor"="scale factor", "Scale"="Scale") -> (w776:cluster{"scale factor":dbl, "Scale":bool})
        n351 = Bundle By Name(cluster=T8 {"Draw"=TRUE, "Target"={"x"=0.0, "y"=0.0}, "Size"={"x"=20.0, "y"=20.0}, "Angle"=0.0, "Color"=1250067, "Thickness"=0, "CrosshairLabel"=""} ("Image Process.Crosshair IN"), "Draw"="draw Xhair", "Size"=w760, "Target.x"="Target.X::1", "Target.y"="Target.Y::1", "Color"="Crosshair\nColor", "Thickness"="Crosshair Thickness", "CrosshairLabel"="Crosshair.Label1::1") -> (w738:T8)
        n352 = property on="Image (IMAQ)" class="ImageControl"() -> ("ROI"=w763:T17)  [unwired: 2 in, 2 out]
        n353 = property on="2ndmomW0x::1" class="DigNum (strict)"() -> ("Value"=w757:dbl)  [unwired: 2 in, 2 out]
        n354 = property on="2ndmomW0y::1" class="DigNum (strict)"() -> ("Value"=w756:dbl)  [unwired: 2 in, 2 out]
        n355 = property on="2ndmomW0x45::1" class="DigNum (strict)"() -> ("Value"=w755:dbl)  [unwired: 2 in, 2 out]
        n356 = property on="2ndmomW0y45::1" class="DigNum (strict)"() -> ("Value"=w754:dbl)  [unwired: 2 in, 2 out]
        n357 = Unbundle By Name("Overlay\nCentroid") -> ("draw Xhair 2"=w748:bool, "Size x"=w751:dbl, "Size y"=w750:dbl, "# images to average"=w746:i32, "Centroid \nOverlay Color"=w745:u32)
        n358 = Bundle By Name(cluster=T14 {"2ndmomW0y45::1"=0.0, "2ndmomW0x45::1"=0.0, "2ndmomW0y::1"=0.0, "2ndmomW0x::1"=0.0} ("Image Analysis.variables"), "2ndmomW0x::1"=w757, "2ndmomW0y45::1"=w756, "2ndmomW0x45::1"=w755, "2ndmomW0y::1"=w754) -> (w758:T14)
        n359 = Bundle("Size x"=w751, "Size y"=w750) -> (w747:cluster{"Size x":dbl, "Size y":dbl})  [unwired: 1 in]
        n360 = Bundle By Name(cluster=T13 {"CentroidX array"=[], "CentroidY array"=[], "CentroidX"=0.0, "CentroidY"=0.0, "# images to average"=1250067, "Crosshair"={"Draw"=FALSE, "Target"={"x"=0.0, "y"=0.0}, "Size"={"x"=0.0, "y"=0.0}, "Angle"=0.0, "Color"=0, "Thickness"=0, "CrosshairLabel"=""}} ("Image Process.GUI_centroid overlay"), "Crosshair.Draw"=w748, "Crosshair.Size"=w747, "# images to average"=w746, "Crosshair.Color"=w745, "CentroidX"="centroidx::1", "CentroidY"="centroidy::1") -> (w744:T13)
        n361 = Bundle By Name(cluster=w743, "Image Process.Image"=w765, "Image Process.Crosshair IN"=w738, "Image Process.Autoscale"="Autoscale", "Image Process.Scale"=w776, "Image Process.Lowpass IN"=w772, "Image Analysis.Analysis.IN"=w764, "Image Analysis.Lineout.IN.ROI"=w763, "Image Analysis.variables"=w758, "Image Process.GUI_centroid overlay"=w744, "Image Process.GUI Crosshair"="GUI Crosshair") -> (w781:T23)
      }
      frame "Action: Read Controls 2" {
        # "Crosshair 2"
        n362 = Bundle("Target2.X::1"="Target2.X::1", "Target2.Y::1"="Target2.Y::1") -> (w790:cluster{"Target2.X::1":dbl, "Target2.Y::1":dbl})  [unwired: 1 in]
        n363 = Bundle("Target2Size.X::1"="Target2Size.X::1", "Target2Size.Y::1"="Target2Size.Y::1") -> (w787:T29)  [unwired: 1 in]
        n364 = Bundle By Name(cluster=w795, "Image Process.Crosshair2 IN.Draw"="draw Xhair 2", "Image Process.Crosshair2 IN.Target"=w790, "Image Process.Crosshair2 IN.Size"=w787, "Image Process.Crosshair2 IN.Color"="Crosshair 2\nColor", "Image Process.Crosshair2 IN.Thickness"="Crosshair 2Thickness", "Image Process.Crosshair2 IN.CrosshairLabel"="Crosshair.Label2::1") -> (w794:T23)
      }
      frame "Action: Process Image" {
        # "GUI running average centroid overlay added by Aalhad (18/6/2017)"
        n365 = Unbundle By Name(w810) -> ("Image Analysis.Analysis.OUT.FWHMx (um)"=w798:dbl, "Image Analysis.Analysis.OUT.FWHMy (um)"=w799:dbl, "Image Analysis.variables.2ndmomW0x::1"=w806:dbl, "Image Analysis.variables.2ndmomW0y::1"=w805:dbl, "Image Analysis.variables.2ndmomW0x45::1"=w804:dbl, "Image Analysis.variables.2ndmomW0y45::1"=w803:dbl)
        n366 = Unbundle By Name(w810) -> ("Graph"=w808:dbl[][])
        n367 = local read "meancounts::1"() -> (w801:dbl)
        n368 = Unbundle By Name(w810) -> ("Image Process"=w817:T20, "Image Analysis"=w812:T21)
        n369 = To Double Precision Float(number=w801) -> (double precision float=w802:dbl)
        n370 = Build Array(w798, w799, w806, w805, w804, w803, "maxcounts::1", w802) -> (w809:dbl[])
        n371 = Build Array (concatenate)(w808, w809) -> (→"Chart":dbl[][])
        n372 = call "Process Image.vi"("error in (no error)"=w814, "Image Analysis IN"=w812, "Cluster in"=w817) -> ("error out"=w813:errorcluster, "Image Analysis OUT"=w811:T21, "Cluster out"=w816:T20)  [unwired: 6 in]
        n373 = Bundle By Name(cluster=w810, "Image Process"=w816, "Image Analysis"=w811) -> (w815:T23)
      }
      frame "Action: Display Image" {
        # "Max count before and after image processing is added by Aalhad"
        n374 = Unbundle By Name(w819) -> ("Image Process.Image"=→"Image (IMAQ)":T1, "Image Analysis.Lineout.OUT"=w837:T30, "Image Analysis.Histogram OUT"=w836:T31, "Image Analysis.Analysis.OUT"=w833:cluster{"FWHMx (um)":dbl, "FWHMy (um)":dbl}, "Image Process.Crosshair IN.Draw"=w829:bool, "Image Process.Crosshair IN.Target.x"=w827:dbl, "Image Process.Crosshair IN.Target.y"=w826:dbl, "Max count"=w821:dbl, "Max count before Image Processing"=w820:dbl)
        n375 = case shown="\"After Image Processing\", Default" "Max count" {
          tunnel: [w841 w842] -> w822
          tunnel: w821 -> [w841 _]
          tunnel: w820 -> [_ w842]
          frame "After Image Processing", Default {
          }
          frame "Before Image Processing" {
          }
        }
        "Max Counts" <- w822
        n376 = call-poly <userlib>:"Data Changed__ogtk.vi"("Boolean"=w829) -> ("Changed"=w828:bool)
        n377 = Unbundle By Name(w837) -> ("lineout"=→"lineout":cluster{"x0":sgl, "dx":sgl, "Pixels Line":sgl[]})  [unwired: 1 out]
        n378 = Unbundle By Name(w836) -> ("histogram"=→"histogram":T9, "Mean Value"=→"Mean Value":sgl)  [unwired: 1 out]
        n379 = case shown="True" w828 {
          tunnel: w827 -> [_ w845]
          tunnel: w826 -> [_ w844]
          frame False {
          }
          frame True {
            n380 = Bundle("x"=w845, "y"=w844) -> (w843:cluster{"x":dbl, "y":dbl})  [unwired: 1 in]
            n381 = property on="Image (IMAQ)" class="ImageControl"("Image Center Position"=w843) -> ()  [unwired: 2 in, 2 out]
          }
        }
        n382 = Unbundle By Name(w833) -> ("FWHMx (um)"=→"FWHMx (um)":dbl, "FWHMy (um)"=→"FWHMy (um)":dbl)
        n383 = call "ColorRamp_TS.vi"("max value"=256, "value"=w822) -> ("Color"=w824:u32)  [unwired: 9 in]
        n384 = property on="Max Counts" class="Slide (strict)"("Fill Color"=w824) -> ()  [unwired: 2 in, 2 out]
      }
      frame "Action: Color Table" {
        # "Chech whether user input for color table\nother than Ni pallete"
        # "When user cancels the make new one color table \nthen color table value changed to rainbow"
        n385 = property on="Color table" class="Enum (strict)"() -> ("Strings []"=w850:string[])  [unwired: 2 in, 2 out]
        n386 = Format Into String("Color table") -> (resulting string=w851:string)  [unwired: 3 in, 1 out]
        n387 = call "IMAQ color table presets.vi"("Color table"="Color table") -> ("Make new one cancelled"=w846:bool, "Array"=w855:cluster{"R":u8, "G":u8, "B":u8}[])  [unwired: 9 in]
        n388 = Search 1D Array(1D array=w850, element=w851) -> (index of element=w848:i32)  [unwired: 1 in]
        n389 = Greater Or Equal?(x=w848, y=5) -> (x >= y?=w849:bool)
        n390 = case shown="True" w849 {
          tunnel: w855 -> [_ w864]
          tunnel: "Color table" -> [w860 _]
          tunnel: w854 -> [w859 w861]
          tunnel: [w858 w863] -> w853
          tunnel: w846 -> [_ w862]
          frame False {
            n391 = property on="Image (IMAQ)" class="ImageControl"(error in=w859, "Palette Type"=w860) -> (error out=w858:errorcluster)  [unwired: 1 in, 1 out]
          }
          frame True {
            w865 = u32 5 items=["Grayscale", "Binary", "Gradient", "Rainbow", "Temperature", "User Defined"] ("Palette:Palette Type")
            n392 = case shown="True" w862 {
              tunnel: w861 -> [_ w866]
              frame False {
              }
              frame True {
                n393 = property on="Color table" class="Enum (strict)"(error in=w866, "Val(Sgnl)"=image_color_table_presets."Rainbow" ("Value (Signaling)")) -> ()  [unwired: 1 in, 2 out]
              }
            }
            n394 = property on="Image (IMAQ)" class="ImageControl"(error in=w861, "Palette Type"=w865, "User Palette"=w864) -> (error out=w863:errorcluster)  [unwired: 1 in, 1 out]
          }
        }
      }
      frame "Action: Beep If Saturation" {
        n395 = Unbundle By Name(w871) -> ("Image Analysis.Lineout.OUT.Max Counts.Max"=w870:sgl)
        n396 = call "Beep if saturation.vi"("error in"=w869, "Sat Level"="Sat Level", "Beep If Sat."="Beep If Sat.", "Max"=w870) -> ("error out"=w868:errorcluster)  [unwired: 7 in]
      }
      frame "Action: Hide Controls" {
        w891 = u32 0 items=["Visible", "Hidden", "Hidden, Use WindTools Palette"] ("ROI Tools Visible")
        # "As the user hide and show controls we need to resize the \npanel by adding and subtracting certain number to \"Right\" FP Bounds. The minimum pane size should be set as per the below: \n\n1. Left - Right = Width (877)\n2. Top - Bottom = Height (500)"
        # "As per the tab size splitter position is set"
        # "Hide splitter"
        n397 = Unbundle By Name(w888) -> ("Image Data.Image Area"=w901:cluster{"Width":u32, "Height":u32})
        n398 = Not(x="Hide controls") -> (.not. x?=w876:bool)
        n399 = local write "Hide controls"(w876) -> ()
        n400 = case shown="True" w876 {
          tunnel: [372 ("Position:Left") w911] -> w900
          tunnel: w878 -> [w909 w913]
          tunnel: [w908 w912] -> w877
          frame False {
            w910 = u32 12369084 ("Color")
            n401 = property on="Splitter" class="Splitter"(error in=w909, "FGColor"=w910, "BGColor"=w910) -> (error out=w908:errorcluster)  [unwired: 1 in, 1 out]
          }
          frame True {
            w911 = 2 ("Position:Left")
            w914 = u32 14869218 ("Color")
            n402 = property on="Splitter" class="Splitter"("Position"=w911) -> ()  [unwired: 2 in, 2 out]
            n403 = property on="Splitter" class="Splitter"(error in=w913, "FGColor"=w914, "BGColor"=w914) -> (error out=w912:errorcluster)  [unwired: 1 in, 1 out]
          }
        }
        n404 = property on="Image (IMAQ)" class="ImageControl"() -> ("ROI Tools Visible"=w892:u32)  [unwired: 2 in, 2 out]
        n405 = property class="VI"(error in=w877) -> (error out=w883:errorcluster, "Front Panel.WinBounds"=w885:T22)  [unwired: 1 in, 1 out]
        n406 = Equal?(x=w892, y=w891) -> (x = y?=w890:bool)
        n407 = Unbundle By Name(w885) -> ("Right"=w882:i16)
        n408 = property on="Image (IMAQ)" class="ImageControl"(error in=w883, "Image Area Size"=w901, "Zoom to Fit Mode"=FALSE) -> (error out=w897:errorcluster)  [unwired: 1 in, 1 out]
        n409 = Select(t=420 ("Position:Left"), s=w890, f=390 ("Position:Left")) -> (s? t:f=w881:i32)
        n410 = Subtract(x=w882, y=w881) -> (x-y=w895:i32)
        n411 = Add(x=w881, y=w882) -> (x+y=w894:i32)
        n412 = Select(t=w895, s=w876, f=w894) -> (s? t:f=w893:i32)
        n413 = invoke on="Image (IMAQ)" class="ImageControl" method="FitControlToPane"(error in=w897) -> (error out=w884:errorcluster)  [unwired: 2 in, 2 out]
        n414 = Bundle By Name(cluster=w885, "Right"=w893) -> (w896:T22)
        n415 = property class="VI"(error in=w884, "Front Panel.WinBounds"=w896) -> (error out=w875:errorcluster)  [unwired: 1 in, 1 out]
        n416 = case shown="False" w876 {
          tunnel: w900 -> [w905 _]
          tunnel: [w904 w906] -> w879
          tunnel: w875 -> [w903 w906]
          frame False {
            n417 = property on="Splitter" class="Splitter"(error in=w903, "Position"=w905) -> (error out=w904:errorcluster)  [unwired: 1 in, 1 out]
          }
          frame True {
          }
        }
        n418 = invoke on="Image (IMAQ)" class="ImageControl" method="FitControlToPane"(error in=w879) -> (error out=w880:errorcluster)  [unwired: 2 in, 2 out]
        n419 = call <vilib>:"Add State(s) to Queue__jki_lib_state_machine.vi"("State(s) in (\"\")"=w899) -> ("States Out"=w898:string)  [unwired: 14 in]
      }
    }
  }
